vi "6层电梯.vi"() -> ()   [LabVIEW 2014]
panel:
  out "超重灯":bool
  in  "重量":dbl
  in  "常开":bool
  in  "开":bool
  in  "关":bool
  in  "电梯快行":bool
  in  "5下":bool
  out "6楼显示":string
  in  "6下":bool
  out "6楼门":bool
  in  "6楼":bool
  out "电梯内显示":string
  out "5楼显示":string
  out "4楼显示":string
  out "3楼显示":string
  out "2楼显示":string
  out "1楼显示":string
  in  "?":bool
  out "上/下":i32
  in  "2下":bool
  in  "3下":bool
  in  "4下":bool
  in  "3上":bool
  in  "1上":bool
  in  "2上":bool
  in  "4上":bool
  in  "5上":bool
  in  "电梯门":bool
  in  "3楼":bool
  in  "1楼":bool
  in  "2楼":bool
  in  "4楼":bool
  in  "5楼":bool
  out "5楼门":bool
  out "4楼门":bool
  out "3楼门":bool
  out "2楼门":bool
  out "1楼门":bool
  # "门开6秒后检测重量，大于1000则\n不会关门，需手动修改"
  # "模仿人为用物品遮挡电梯门，导致电梯不能\n关门执行下一步动作，常开点亮需手动熄灭\n使电梯门关。"
  # "在门打开期间\n开、关禁止同时点亮，会造成程序运行错误"
  # "点亮开按钮，延时5S关门"
  # "点亮关按钮，门立即关闭"
  # "点亮灯电梯快速运行\n熄灭灯慢速运行"
  # "电梯内按钮"
  # "电梯外部按钮"
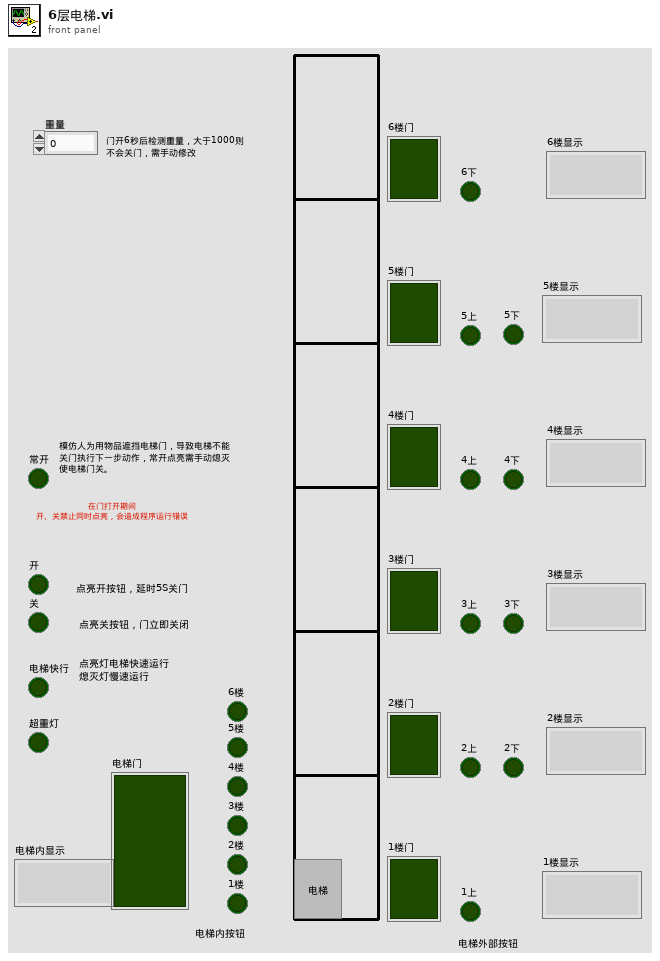
[diagram p1: front panel]
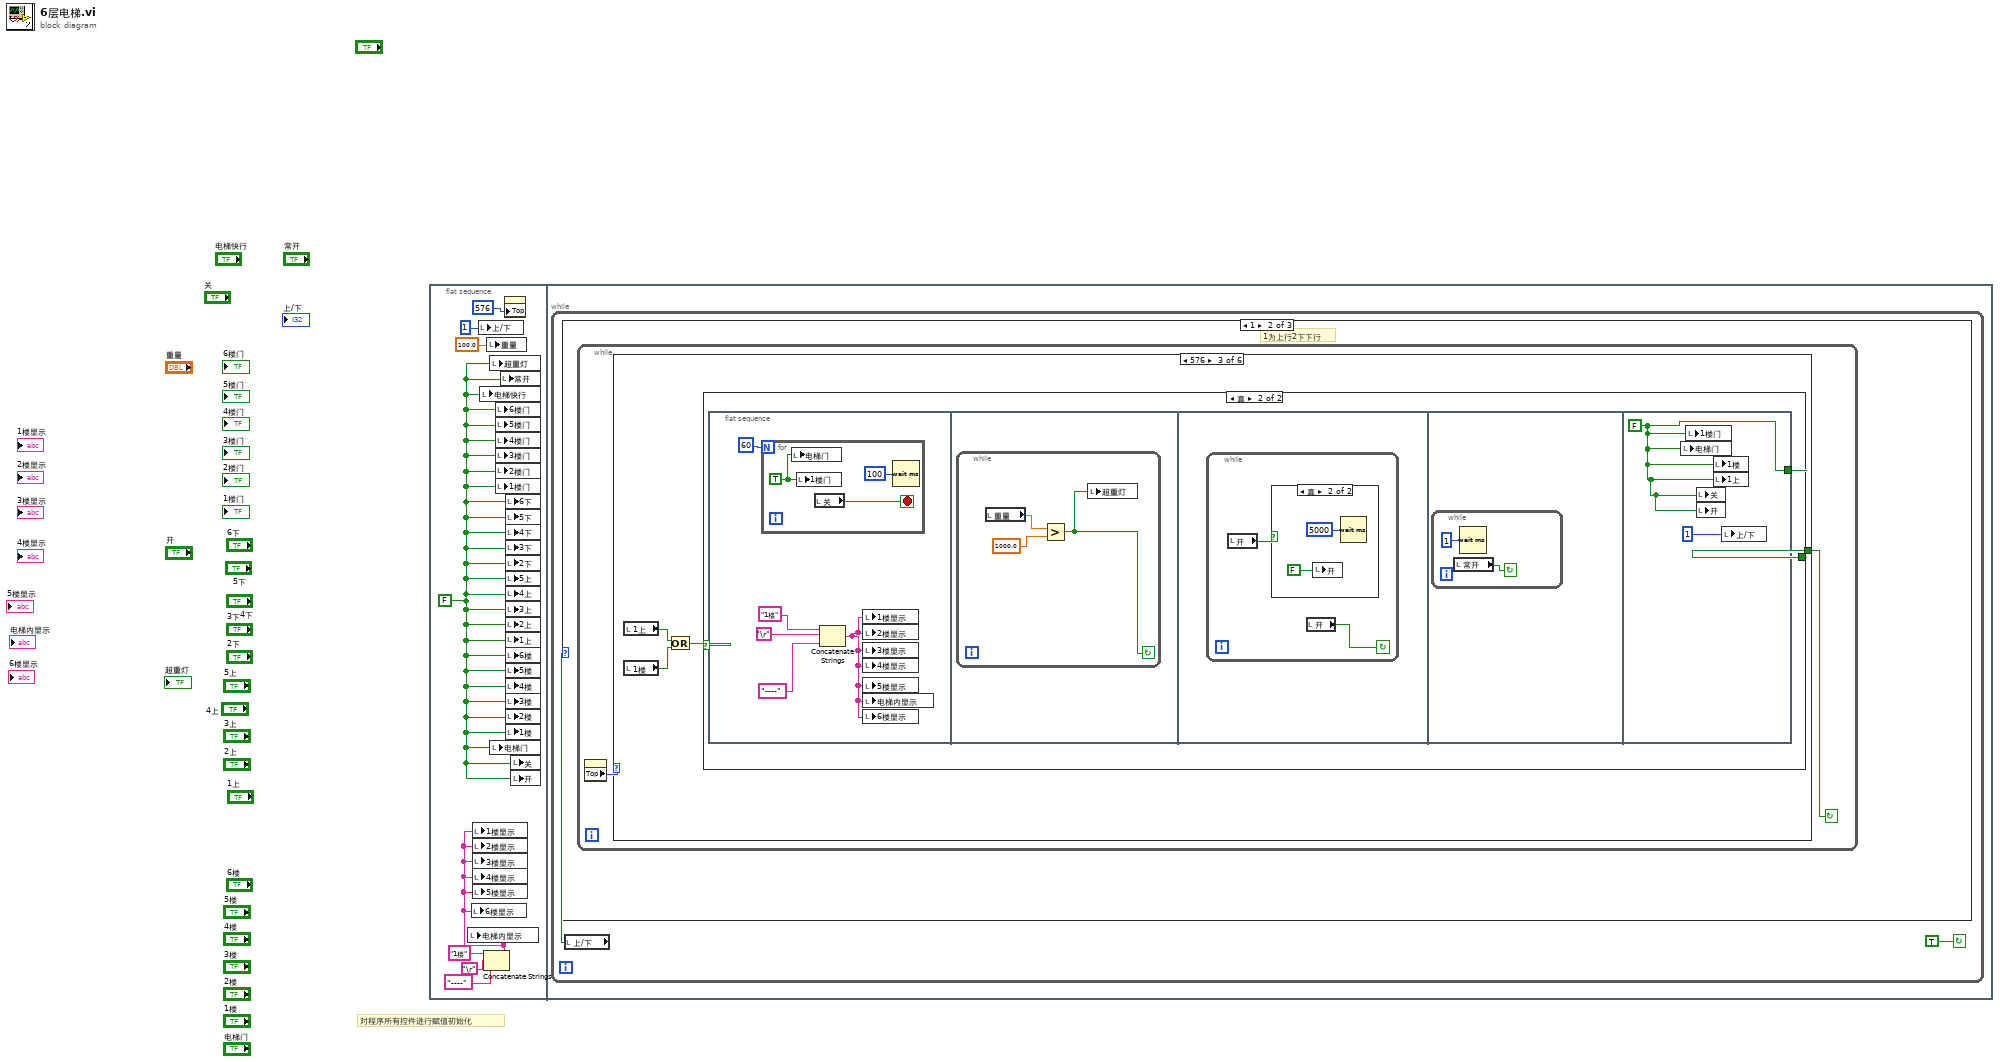
[diagram p0: block diagram]
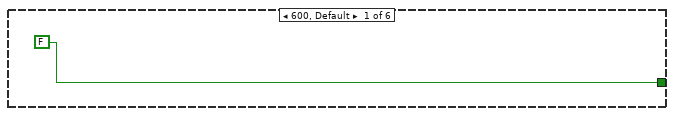
[diagram p3: hidden frame]
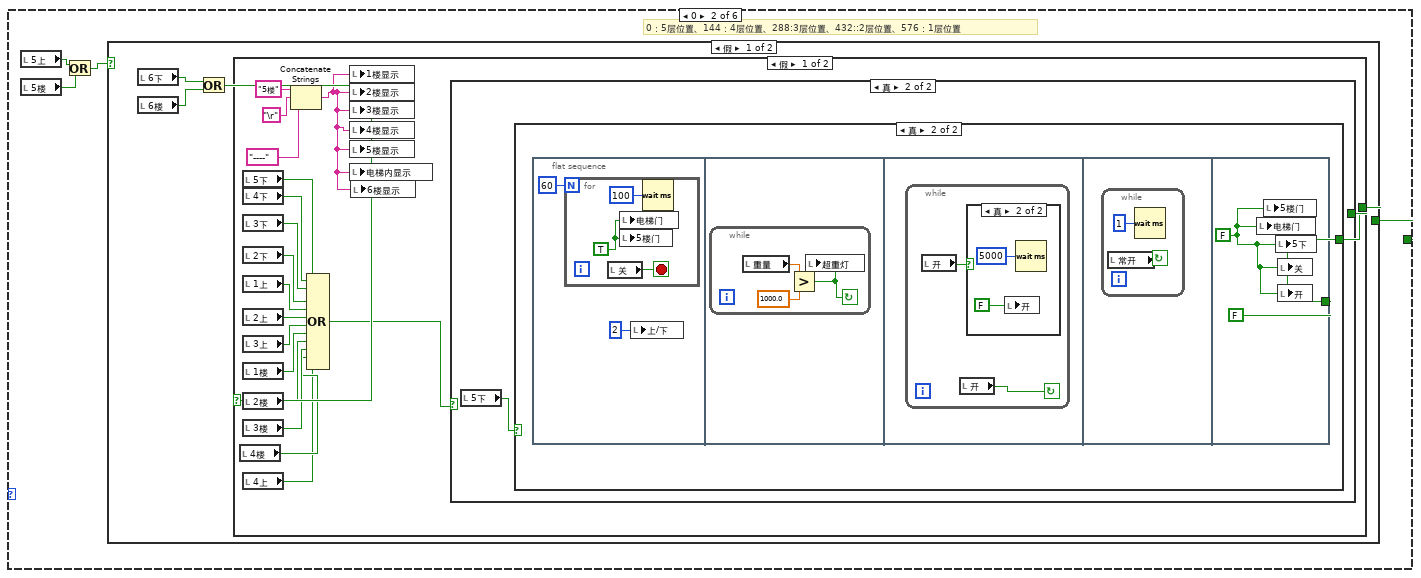
[diagram p4: hidden frame]
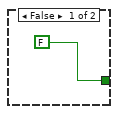
[diagram p5: hidden frame]
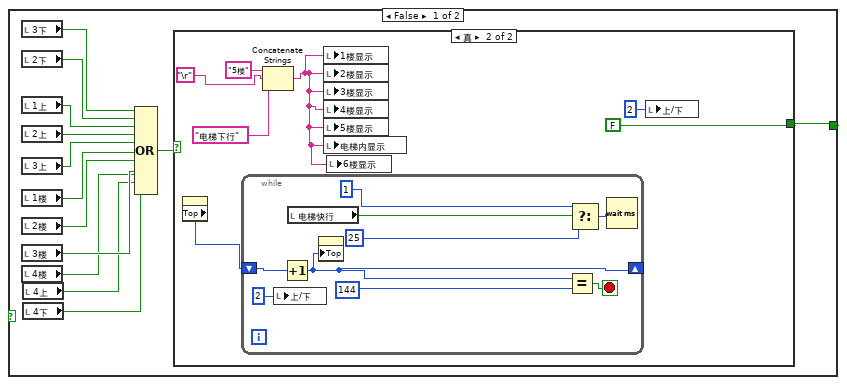
[diagram p6: hidden frame]
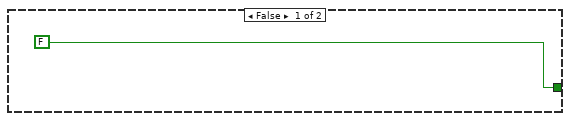
[diagram p7: hidden frame]
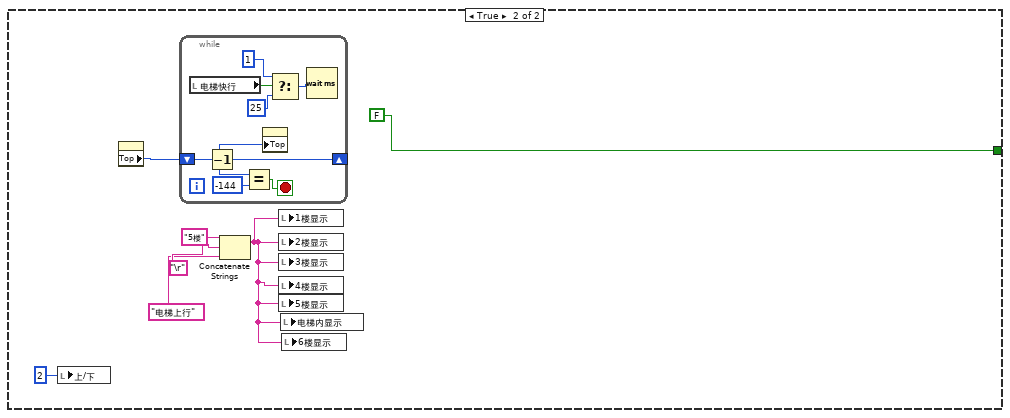
[diagram p9: hidden frame]
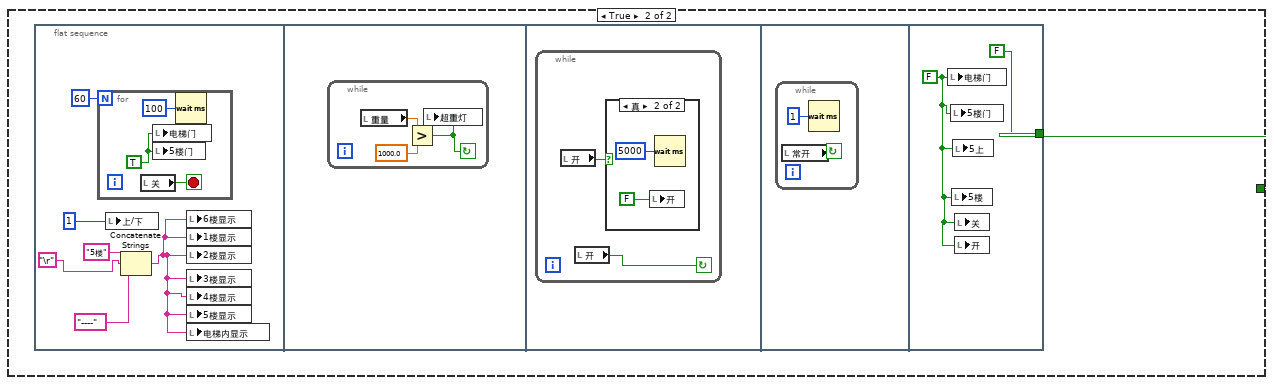
[diagram p10: hidden frame]
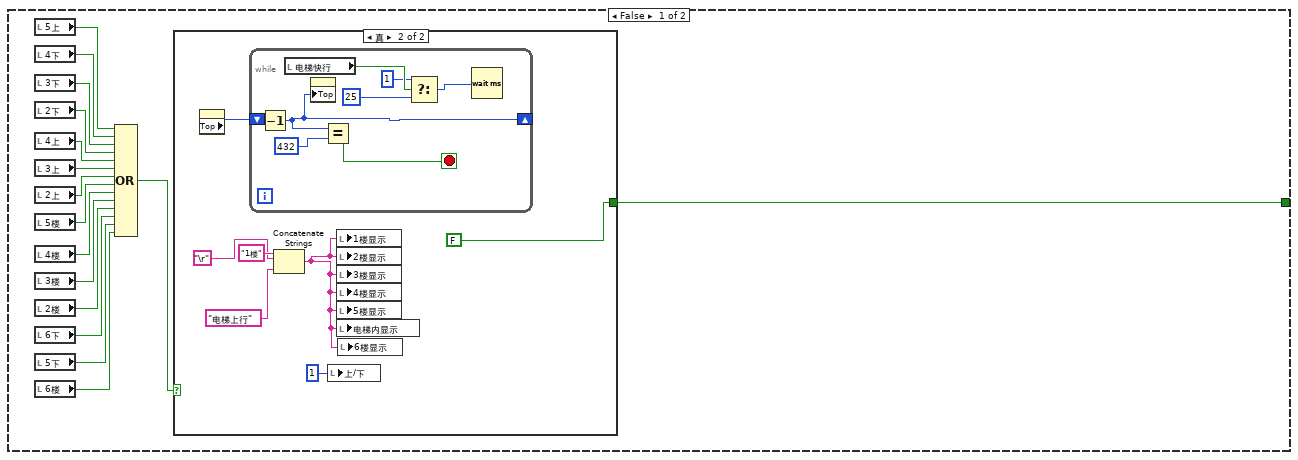
[diagram p12: hidden frame]
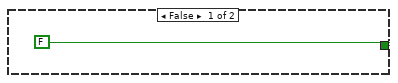
[diagram p13: hidden frame]
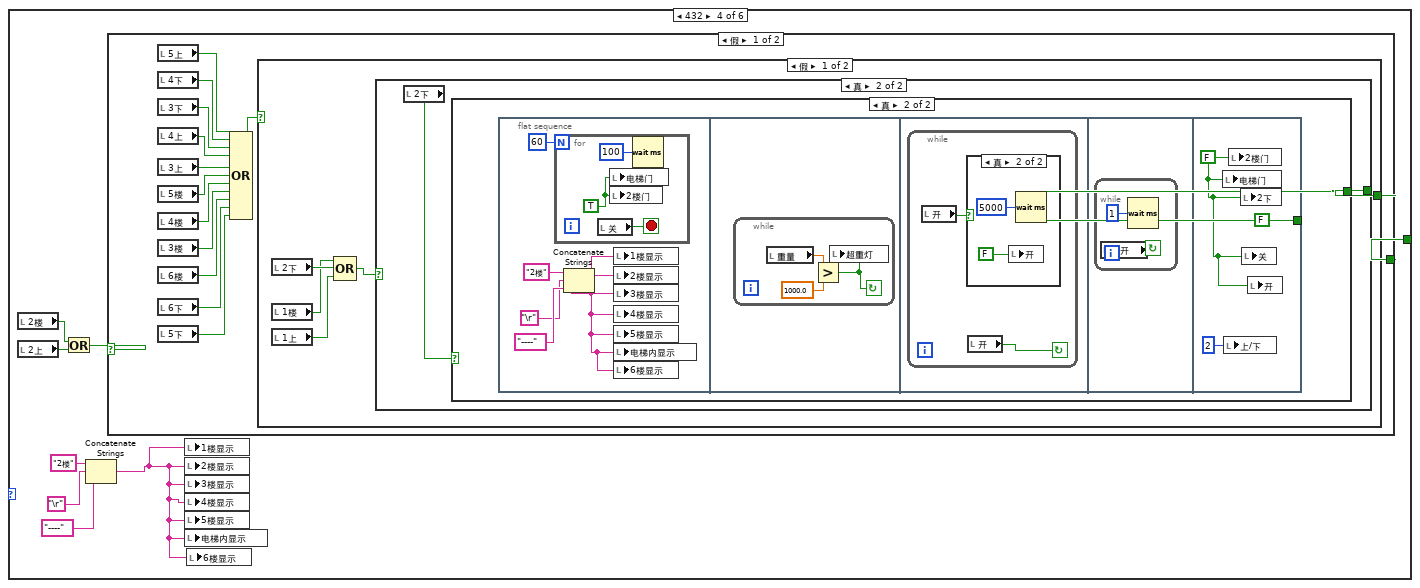
[diagram p15: hidden frame]
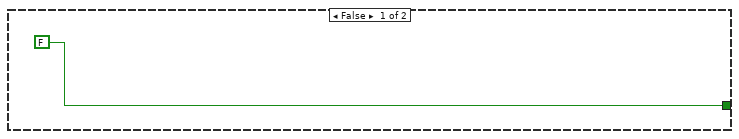
[diagram p16: hidden frame]
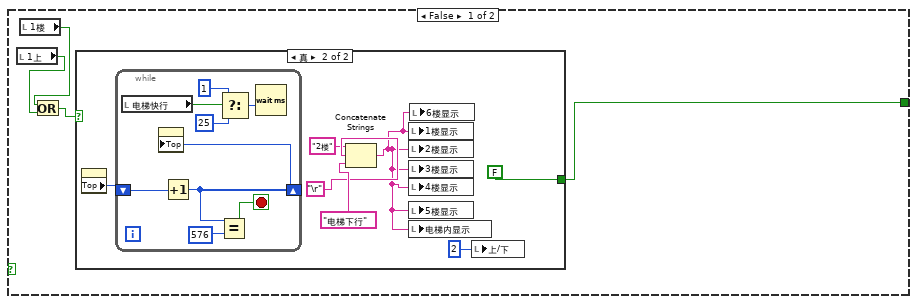
[diagram p17: hidden frame]
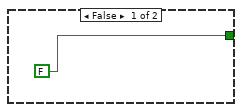
[diagram p18: hidden frame]
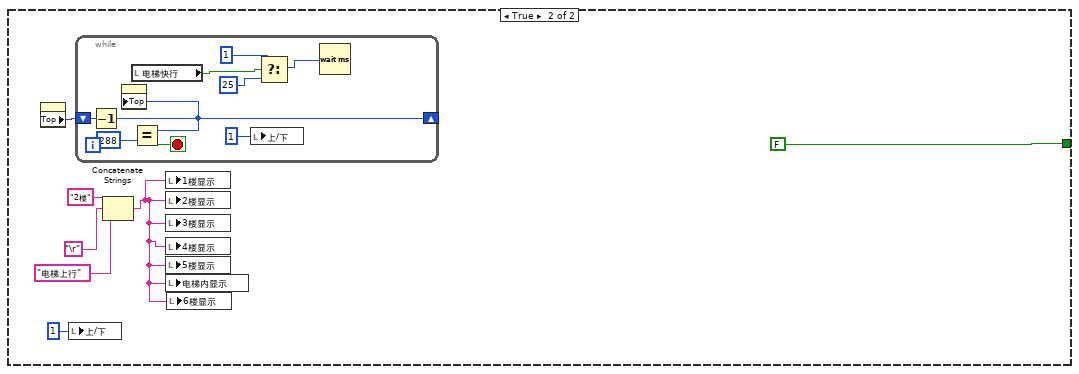
[diagram p20: hidden frame]
diagram:
  # "对程序所有控件进行赋值初始化"
  n1 = flat-sequence {
    frame #0 {
      w1 = FALSE
      n2 = local write "上/下"(1 ("上/下")) -> ()
      n3 = local write "电梯快行"(w1) -> ()
      n4 = Concatenate Strings("1楼" ("字符串"), "\r", "----" ("字符串")) -> (w3:string)
      n5 = local write "电梯内显示"(w3) -> ()
      n6 = local write "6楼显示"(w3) -> ()
      n7 = local write "1楼显示"(w3) -> ()
      n8 = local write "2楼显示"(w3) -> ()
      n9 = local write "3楼显示"(w3) -> ()
      n10 = local write "4楼显示"(w3) -> ()
      n11 = local write "5楼显示"(w3) -> ()
      n12 = local write "重量"(100.0 ("重量")) -> ()
      n13 = local write "超重灯"(w1) -> ()
      n14 = local write "电梯门"(w1) -> ()
      n15 = local write "6楼门"(w1) -> ()
      n16 = local write "5楼门"(w1) -> ()
      n17 = local write "4楼门"(w1) -> ()
      n18 = local write "3楼门"(w1) -> ()
      n19 = local write "2楼门"(w1) -> ()
      n20 = local write "1楼门"(w1) -> ()
      n21 = local write "常开"(w1) -> ()
      n22 = property class="Bool"("Top"=576 ("位置:置顶")) -> ()  [unwired: 2 in, 2 out]
      n23 = local write "6下"(w1) -> ()
      n24 = local write "5下"(w1) -> ()
      n25 = local write "4下"(w1) -> ()
      n26 = local write "3下"(w1) -> ()
      n27 = local write "2下"(w1) -> ()
      n28 = local write "5上"(w1) -> ()
      n29 = local write "4上"(w1) -> ()
      n30 = local write "3上"(w1) -> ()
      n31 = local write "2上"(w1) -> ()
      n32 = local write "1上"(w1) -> ()
      n33 = local write "6楼"(w1) -> ()
      n34 = local write "5楼"(w1) -> ()
      n35 = local write "4楼"(w1) -> ()
      n36 = local write "3楼"(w1) -> ()
      n37 = local write "2楼"(w1) -> ()
      n38 = local write "1楼"(w1) -> ()
      n39 = local write "关"(w1) -> ()
      n40 = local write "开"(w1) -> ()
    }
    frame #1 {
      n41 = while {
        stop <- TRUE continue-if-true
        n42 = local read "上/下"() -> (w10:i32)
        n43 = case shown="1" w10 {
          frame 0, Default {
          }
          frame 1 {
            # "1为上行2下下行"
            n44 = while {
              stop <- w12 continue-if-true
              n45 = property class="Bool"() -> ("Top"=w11:i32)  [unwired: 2 in, 2 out]
              n46 = case shown="576" w11 {
                tunnel: [FALSE w14 w126 w186 w286 w390] -> w12
                frame 600, Default {
                }
                frame 0 {
                  # "0：5层位置、144：4层位置、288:3层位置、432::2层位置、576：1层位置"
                  n47 = local read "5上"() -> (w15:bool)
                  n48 = local read "5楼"() -> (w16:bool)
                  n49 = Or(x=w15, y=w16) -> (x .or. y?=w17:bool)
                  n50 = case shown="假" w17 {
                    tunnel: [w21 w105] -> w14
                    frame False {
                      n51 = local read "6下"() -> (w19:bool)
                      n52 = local read "6楼"() -> (w18:bool)
                      n53 = Or(x=w19, y=w18) -> (x .or. y?=w20:bool)
                      n54 = case shown="假" w20 {
                        tunnel: [w39 FALSE] -> w21
                        frame False {
                          n55 = local read "4楼"() -> (w23:bool)
                          n56 = local read "5下"() -> (w25:bool)
                          n57 = local read "4下"() -> (w35:bool)
                          n58 = local read "3下"() -> (w34:bool)
                          n59 = local read "2下"() -> (w33:bool)
                          n60 = local read "1上"() -> (w32:bool)
                          n61 = local read "2上"() -> (w31:bool)
                          n62 = local read "3上"() -> (w30:bool)
                          n63 = local read "1楼"() -> (w29:bool)
                          n64 = local read "2楼"() -> (w28:bool)
                          n65 = local read "3楼"() -> (w27:bool)
                          n66 = local read "4上"() -> (w22:bool)
                          n67 = Concatenate Strings("5楼" ("字符串"), "\r", "----" ("字符串")) -> (w24:string)
                          n68 = Compound Arithmetic op=OR(w25, w35, w34, w33, w32, w31, w30, w29, w28, w27, w23, w22) -> (w26:bool)
                          n69 = local write "1楼显示"(w24) -> ()
                          n70 = local write "2楼显示"(w24) -> ()
                          n71 = local write "3楼显示"(w24) -> ()
                          n72 = local write "4楼显示"(w24) -> ()
                          n73 = local write "5楼显示"(w24) -> ()
                          n74 = local write "电梯内显示"(w24) -> ()
                          n75 = local write "6楼显示"(w24) -> ()
                          n76 = case shown="真" w26 {
                            tunnel: [FALSE w42] -> w39
                            frame False {
                            }
                            frame True {
                              n77 = local read "5下"() -> (w41:bool)
                              n78 = case shown="真" w41 {
                                tunnel: [w46 w73] -> w42
                                frame False {
                                n79 = local read "3下"() -> (w55:bool)
                                n80 = local read "2下"() -> (w54:bool)
                                n81 = local read "1上"() -> (w53:bool)
                                n82 = local read "2上"() -> (w52:bool)
                                n83 = local read "3上"() -> (w51:bool)
                                n84 = local read "1楼"() -> (w50:bool)
                                n85 = local read "2楼"() -> (w49:bool)
                                n86 = local read "3楼"() -> (w48:bool)
                                n87 = local read "4楼"() -> (w45:bool)
                                n88 = local read "4上"() -> (w44:bool)
                                n89 = local read "4下"() -> (w43:bool)
                                n90 = Compound Arithmetic op=OR(w55, w54, w53, w52, w51, w50, w49, w48, w45, w44, w43) -> (w47:bool)
                                n91 = case shown="真" w47 {
                                tunnel: [FALSE FALSE] -> w46
                                frame False {
                                }
                                frame True {
                                n92 = property class="Bool"() -> ("Top"=w63:i32)  [unwired: 2 in, 2 out]
                                n93 = while {
                                shift-right: [w70] -> _
                                shift-left: w63 -> [w72]
                                stop <- w71 stop-if-true
                                n94 = local write "上/下"(2 ("上/下")) -> ()
                                n95 = Increment(x=w72) -> (x+1=w70:i32)
                                n96 = local read "电梯快行"() -> (w66:bool)
                                n97 = property class="Bool"("Top"=w70) -> ()  [unwired: 2 in, 2 out]
                                n98 = Equal?(x=w70, y=144) -> (x = y?=w71:bool)
                                n99 = Select(t=u32 1, s=w66, f=u32 25) -> (s? t:f=w67:u32)
                                n100 = Wait (ms)(milliseconds to wait=w67) -> ()  [unwired: 1 out]
                                }
                                n101 = Concatenate Strings("5楼" ("字符串"), "\r", "电梯下行" ("字符串")) -> (w57:string)
                                n102 = local write "1楼显示"(w57) -> ()
                                n103 = local write "2楼显示"(w57) -> ()
                                n104 = local write "3楼显示"(w57) -> ()
                                n105 = local write "4楼显示"(w57) -> ()
                                n106 = local write "5楼显示"(w57) -> ()
                                n107 = local write "电梯内显示"(w57) -> ()
                                n108 = local write "6楼显示"(w57) -> ()
                                n109 = local write "上/下"(2 ("上/下")) -> ()
                                }
                                }
                                }
                                frame True {
                                n110 = flat-sequence {
                                tunnel: [FALSE] -> w73
                                frame #0 {
                                n111 = for {
                                N: 60 -> [_]
                                stop <- w76 stop-if-true
                                w78 = TRUE ("1楼门")
                                n112 = local read "关"() -> (w76:bool)
                                n113 = local write "电梯门"(w78) -> ()
                                n114 = local write "5楼门"(w78) -> ()
                                n115 = Wait (ms)(milliseconds to wait=u32 100 ("等待时间（毫秒）")) -> ()  [unwired: 1 out]
                                }
                                n116 = local write "上/下"(2 ("上/下")) -> ()
                                }
                                frame #1 {
                                n117 = while {
                                stop <- w79 continue-if-true
                                n118 = local read "重量"() -> (w81:dbl)
                                n119 = Greater?(x=w81, y=1000.0 ("x")) -> (0:w79:bool)
                                n120 = local write "超重灯"(w79) -> ()
                                }
                                }
                                frame #2 {
                                n121 = while {
                                stop <- w82 continue-if-true
                                n122 = local read "开"() -> (w83:bool)
                                n123 = local read "开"() -> (w82:bool)
                                n124 = case shown="真" w83 {
                                frame False {
                                }
                                frame True {
                                n125 = local write "开"(FALSE ("常开")) -> ()
                                n126 = Wait (ms)(milliseconds to wait=u32 5000 ("等待时间（毫秒）")) -> ()  [unwired: 1 out]
                                }
                                }
                                }
                                }
                                frame #3 {
                                n127 = while {
                                stop <- w87 continue-if-true
                                n128 = local read "常开"() -> (w87:bool)
                                n129 = Wait (ms)(milliseconds to wait=u32 1 ("等待时间（毫秒）")) -> ()  [unwired: 1 out]
                                }
                                }
                                frame #4 {
                                w88 = FALSE ("2楼门")
                                n130 = local write "电梯门"(w88) -> ()
                                n131 = local write "5楼门"(w88) -> ()
                                n132 = local write "5下"(w88) -> ()
                                n133 = local write "关"(w88) -> ()
                                n134 = local write "开"(w88) -> ()
                                }
                                }
                                }
                              }
                            }
                          }
                        }
                        frame True {
                          n135 = local write "上/下"(2 ("上/下")) -> ()
                          n136 = property class="Bool"() -> ("Top"=w90:i32)  [unwired: 2 in, 2 out]
                          n137 = while {
                            shift-right: [w103] -> _
                            shift-left: w90 -> [w101]
                            stop <- w104 stop-if-true
                            n138 = local read "电梯快行"() -> (w99:bool)
                            n139 = Decrement(x=w101) -> (x-1=w103:i32)
                            n140 = Equal?(x=w103, y=-144) -> (x = y?=w104:bool)
                            n141 = property class="Bool"("Top"=w103) -> ()  [unwired: 2 in, 2 out]
                            n142 = Select(t=u32 1, s=w99, f=u32 25) -> (s? t:f=w100:u32)
                            n143 = Wait (ms)(milliseconds to wait=w100) -> ()  [unwired: 1 out]
                          }
                          n144 = Concatenate Strings("5楼" ("字符串"), "\r", "电梯上行" ("字符串")) -> (w94:string)
                          n145 = local write "1楼显示"(w94) -> ()
                          n146 = local write "2楼显示"(w94) -> ()
                          n147 = local write "3楼显示"(w94) -> ()
                          n148 = local write "4楼显示"(w94) -> ()
                          n149 = local write "5楼显示"(w94) -> ()
                          n150 = local write "电梯内显示"(w94) -> ()
                          n151 = local write "6楼显示"(w94) -> ()
                        }
                      }
                    }
                    frame True {
                      n152 = flat-sequence {
                        tunnel: [FALSE] -> w105
                        frame #0 {
                          n153 = for {
                            N: 60 -> [_]
                            stop <- w112 stop-if-true
                            w114 = TRUE ("1楼门")
                            n154 = local read "关"() -> (w112:bool)
                            n155 = local write "电梯门"(w114) -> ()
                            n156 = local write "5楼门"(w114) -> ()
                            n157 = Wait (ms)(milliseconds to wait=u32 100 ("等待时间（毫秒）")) -> ()  [unwired: 1 out]
                          }
                          n158 = local write "上/下"(1 ("上/下")) -> ()
                          n159 = Concatenate Strings("5楼" ("字符串"), "\r", "----" ("字符串")) -> (w107:string)
                          n160 = local write "6楼显示"(w107) -> ()
                          n161 = local write "1楼显示"(w107) -> ()
                          n162 = local write "2楼显示"(w107) -> ()
                          n163 = local write "3楼显示"(w107) -> ()
                          n164 = local write "4楼显示"(w107) -> ()
                          n165 = local write "5楼显示"(w107) -> ()
                          n166 = local write "电梯内显示"(w107) -> ()
                        }
                        frame #1 {
                          n167 = while {
                            stop <- w115 continue-if-true
                            n168 = local read "重量"() -> (w117:dbl)
                            n169 = Greater?(x=w117, y=1000.0 ("x")) -> (0:w115:bool)
                            n170 = local write "超重灯"(w115) -> ()
                          }
                        }
                        frame #2 {
                          n171 = while {
                            stop <- w118 continue-if-true
                            n172 = local read "开"() -> (w119:bool)
                            n173 = local read "开"() -> (w118:bool)
                            n174 = case shown="真" w119 {
                              frame False {
                              }
                              frame True {
                                n175 = local write "开"(FALSE ("常开")) -> ()
                                n176 = Wait (ms)(milliseconds to wait=u32 5000 ("等待时间（毫秒）")) -> ()  [unwired: 1 out]
                              }
                            }
                          }
                        }
                        frame #3 {
                          n177 = while {
                            stop <- w123 continue-if-true
                            n178 = local read "常开"() -> (w123:bool)
                            n179 = Wait (ms)(milliseconds to wait=u32 1 ("等待时间（毫秒）")) -> ()  [unwired: 1 out]
                          }
                        }
                        frame #4 {
                          w124 = FALSE ("电梯门")
                          n180 = local write "电梯门"(w124) -> ()
                          n181 = local write "5楼门"(w124) -> ()
                          n182 = local write "5楼"(w124) -> ()
                          n183 = local write "5上"(w124) -> ()
                          n184 = local write "关"(w124) -> ()
                          n185 = local write "开"(w124) -> ()
                        }
                      }
                    }
                  }
                }
                frame 576 {
                  n186 = local read "1上"() -> (w129:bool)
                  n187 = local read "1楼"() -> (w128:bool)
                  n188 = Or(x=w129, y=w128) -> (x .or. y?=w127:bool)
                  n189 = case shown="真" w127 {
                    tunnel: [w134 w162] -> w126
                    frame False {
                      n190 = local read "5上"() -> (w145:bool)
                      n191 = local read "4下"() -> (w144:bool)
                      n192 = local read "3下"() -> (w143:bool)
                      n193 = local read "2下"() -> (w142:bool)
                      n194 = local read "4上"() -> (w141:bool)
                      n195 = local read "3上"() -> (w140:bool)
                      n196 = local read "2上"() -> (w139:bool)
                      n197 = local read "5楼"() -> (w138:bool)
                      n198 = local read "4楼"() -> (w137:bool)
                      n199 = local read "3楼"() -> (w136:bool)
                      n200 = local read "2楼"() -> (w133:bool)
                      n201 = local read "6下"() -> (w132:bool)
                      n202 = local read "5下"() -> (w131:bool)
                      n203 = local read "6楼"() -> (w130:bool)
                      n204 = Compound Arithmetic op=OR(w145, w144, w143, w142, w141, w140, w139, w138, w137, w136, w133, w132, w131, w130) -> (w135:bool)
                      n205 = case shown="真" w135 {
                        tunnel: [FALSE FALSE] -> w134
                        frame False {
                        }
                        frame True {
                          n206 = property class="Bool"() -> ("Top"=w150:i32)  [unwired: 2 in, 2 out]
                          n207 = while {
                            shift-right: [w159] -> _
                            shift-left: w150 -> [w161]
                            stop <- w160 stop-if-true
                            n208 = Decrement(x=w161) -> (x-1=w159:i32)
                            n209 = local read "电梯快行"() -> (w155:bool)
                            n210 = property class="Bool"("Top"=w159) -> ()  [unwired: 2 in, 2 out]
                            n211 = Equal?(x=w159, y=432) -> (x = y?=w160:bool)
                            n212 = Select(t=u32 1, s=w155, f=u32 25 ("等待时间（毫秒）")) -> (s? t:f=w157:u32)
                            n213 = Wait (ms)(milliseconds to wait=w157) -> ()  [unwired: 1 out]
                          }
                          n214 = Concatenate Strings("1楼" ("字符串"), "\r", "电梯上行" ("字符串")) -> (w147:string)
                          n215 = local write "上/下"(1 ("上/下")) -> ()
                          n216 = local write "1楼显示"(w147) -> ()
                          n217 = local write "2楼显示"(w147) -> ()
                          n218 = local write "3楼显示"(w147) -> ()
                          n219 = local write "4楼显示"(w147) -> ()
                          n220 = local write "5楼显示"(w147) -> ()
                          n221 = local write "电梯内显示"(w147) -> ()
                          n222 = local write "6楼显示"(w147) -> ()
                        }
                      }
                    }
                    frame True {
                      n223 = flat-sequence {
                        tunnel: [w180] -> w162
                        frame #0 {
                          n224 = for {
                            N: 60 -> [_]
                            stop <- w168 stop-if-true
                            w170 = TRUE ("1楼门")
                            n225 = local write "电梯门"(w170) -> ()
                            n226 = local write "1楼门"(w170) -> ()
                            n227 = local read "关"() -> (w168:bool)
                            n228 = Wait (ms)(milliseconds to wait=u32 100 ("等待时间（毫秒）")) -> ()  [unwired: 1 out]
                          }
                          n229 = Concatenate Strings("1楼" ("字符串"), "\r", "----" ("字符串")) -> (w164:string)
                          n230 = local write "1楼显示"(w164) -> ()
                          n231 = local write "2楼显示"(w164) -> ()
                          n232 = local write "3楼显示"(w164) -> ()
                          n233 = local write "4楼显示"(w164) -> ()
                          n234 = local write "5楼显示"(w164) -> ()
                          n235 = local write "电梯内显示"(w164) -> ()
                          n236 = local write "6楼显示"(w164) -> ()
                        }
                        frame #1 {
                          n237 = while {
                            stop <- w171 continue-if-true
                            n238 = local read "重量"() -> (w173:dbl)
                            n239 = Greater?(x=w173, y=1000.0 ("x")) -> (0:w171:bool)
                            n240 = local write "超重灯"(w171) -> ()
                          }
                        }
                        frame #2 {
                          n241 = while {
                            stop <- w174 continue-if-true
                            n242 = local read "开"() -> (w175:bool)
                            n243 = case shown="真" w175 {
                              frame False {
                              }
                              frame True {
                                n244 = local write "开"(FALSE ("常开")) -> ()
                                n245 = Wait (ms)(milliseconds to wait=u32 5000 ("等待时间（毫秒）")) -> ()  [unwired: 1 out]
                              }
                            }
                            n246 = local read "开"() -> (w174:bool)
                          }
                        }
                        frame #3 {
                          n247 = while {
                            stop <- w179 continue-if-true
                            n248 = local read "常开"() -> (w179:bool)
                            n249 = Wait (ms)(milliseconds to wait=u32 1 ("等待时间（毫秒）")) -> ()  [unwired: 1 out]
                          }
                        }
                        frame #4 {
                          w180 = FALSE ("1楼门")
                          n250 = local write "电梯门"(w180) -> ()
                          n251 = local write "1楼门"(w180) -> ()
                          n252 = local write "关"(w180) -> ()
                          n253 = local write "开"(w180) -> ()
                          n254 = local write "1楼"(w180) -> ()
                          n255 = local write "1上"(w180) -> ()
                          n256 = local write "上/下"(1 ("上/下")) -> ()
                        }
                      }
                    }
                  }
                }
                frame 432 {
                  n257 = local read "2楼"() -> (w189:bool)
                  n258 = local read "2上"() -> (w188:bool)
                  n259 = Or(x=w189, y=w188) -> (x .or. y?=w187:bool)
                  n260 = Concatenate Strings("2楼" ("字符串"), "\r", "----" ("字符串")) -> (w182:string)
                  n261 = case shown="假" w187 {
                    tunnel: [w202 w268] -> w186
                    frame False {
                      n262 = local read "5上"() -> (w200:bool)
                      n263 = local read "4下"() -> (w199:bool)
                      n264 = local read "3下"() -> (w198:bool)
                      n265 = local read "4上"() -> (w197:bool)
                      n266 = local read "3上"() -> (w196:bool)
                      n267 = local read "5楼"() -> (w195:bool)
                      n268 = local read "4楼"() -> (w194:bool)
                      n269 = local read "3楼"() -> (w193:bool)
                      n270 = local read "6楼"() -> (w192:bool)
                      n271 = local read "6下"() -> (w191:bool)
                      n272 = local read "5下"() -> (w190:bool)
                      n273 = Compound Arithmetic op=OR(w200, w199, w198, w197, w196, w195, w194, w193, w192, w191, w190) -> (w201:bool)
                      n274 = case shown="假" w201 {
                        tunnel: [w207 FALSE] -> w202
                        frame False {
                          n275 = local read "2下"() -> (w206:bool)
                          n276 = local read "1楼"() -> (w205:bool)
                          n277 = local read "1上"() -> (w204:bool)
                          n278 = Compound Arithmetic op=OR(w205, w206, w204) -> (w203:bool)
                          n279 = case shown="真" w203 {
                            tunnel: [FALSE w210] -> w207
                            frame False {
                            }
                            frame True {
                              n280 = local read "2下"() -> (w209:bool)
                              n281 = case shown="真" w209 {
                                tunnel: [w212 w231] -> w210
                                frame False {
                                n282 = local read "1上"() -> (w213:bool)
                                n283 = local read "1楼"() -> (w214:bool)
                                n284 = Or(x=w214, y=w213) -> (x .or. y?=w211:bool)
                                n285 = case shown="真" w211 {
                                tunnel: [FALSE FALSE] -> w212
                                frame False {
                                }
                                frame True {
                                n286 = property class="Bool"() -> ("Top"=w222:i32)  [unwired: 2 in, 2 out]
                                n287 = while {
                                shift-right: [w228] -> _
                                shift-left: w222 -> [w230]
                                stop <- w229 stop-if-true
                                n288 = local read "电梯快行"() -> (w225:bool)
                                n289 = Increment(x=w230) -> (x+1=w228:i32)
                                n290 = property class="Bool"("Top"=w228) -> ()  [unwired: 2 in, 2 out]
                                n291 = Equal?(x=w228, y=576) -> (x = y?=w229:bool)
                                n292 = Select(t=u32 1, s=w225, f=u32 25 ("等待时间（毫秒）")) -> (s? t:f=w223:u32)
                                n293 = Wait (ms)(milliseconds to wait=w223) -> ()  [unwired: 1 out]
                                }
                                n294 = Concatenate Strings("2楼" ("字符串"), "\r", "电梯下行" ("字符串")) -> (w216:string)
                                n295 = local write "1楼显示"(w216) -> ()
                                n296 = local write "2楼显示"(w216) -> ()
                                n297 = local write "3楼显示"(w216) -> ()
                                n298 = local write "4楼显示"(w216) -> ()
                                n299 = local write "5楼显示"(w216) -> ()
                                n300 = local write "电梯内显示"(w216) -> ()
                                n301 = local write "6楼显示"(w216) -> ()
                                n302 = local write "上/下"(2 ("上/下")) -> ()
                                }
                                }
                                }
                                frame True {
                                n303 = flat-sequence {
                                tunnel: [FALSE] -> w231
                                frame #0 {
                                n304 = for {
                                N: 60 -> [_]
                                stop <- w237 stop-if-true
                                w239 = TRUE ("1楼门")
                                n305 = local read "关"() -> (w237:bool)
                                n306 = local write "电梯门"(w239) -> ()
                                n307 = local write "2楼门"(w239) -> ()
                                n308 = Wait (ms)(milliseconds to wait=u32 100 ("等待时间（毫秒）")) -> ()  [unwired: 1 out]
                                }
                                n309 = Concatenate Strings("2楼" ("字符串"), "\r", "----" ("字符串")) -> (w233:string)
                                n310 = local write "1楼显示"(w233) -> ()
                                n311 = local write "2楼显示"(w233) -> ()
                                n312 = local write "3楼显示"(w233) -> ()
                                n313 = local write "4楼显示"(w233) -> ()
                                n314 = local write "5楼显示"(w233) -> ()
                                n315 = local write "电梯内显示"(w233) -> ()
                                n316 = local write "6楼显示"(w233) -> ()
                                }
                                frame #1 {
                                n317 = while {
                                stop <- w240 continue-if-true
                                n318 = local read "重量"() -> (w242:dbl)
                                n319 = Greater?(x=w242, y=1000.0 ("x")) -> (0:w240:bool)
                                n320 = local write "超重灯"(w240) -> ()
                                }
                                }
                                frame #2 {
                                n321 = while {
                                stop <- w243 continue-if-true
                                n322 = local read "开"() -> (w244:bool)
                                n323 = case shown="真" w244 {
                                frame False {
                                }
                                frame True {
                                n324 = local write "开"(FALSE ("常开")) -> ()
                                n325 = Wait (ms)(milliseconds to wait=u32 5000 ("等待时间（毫秒）")) -> ()  [unwired: 1 out]
                                }
                                }
                                n326 = local read "开"() -> (w243:bool)
                                }
                                }
                                frame #3 {
                                n327 = while {
                                stop <- w248 continue-if-true
                                n328 = local read "常开"() -> (w248:bool)
                                n329 = Wait (ms)(milliseconds to wait=u32 1 ("等待时间（毫秒）")) -> ()  [unwired: 1 out]
                                }
                                }
                                frame #4 {
                                w249 = FALSE ("2楼门")
                                n330 = local write "电梯门"(w249) -> ()
                                n331 = local write "上/下"(2 ("上/下")) -> ()
                                n332 = local write "2楼门"(w249) -> ()
                                n333 = local write "2下"(w249) -> ()
                                n334 = local write "关"(w249) -> ()
                                n335 = local write "开"(w249) -> ()
                                }
                                }
                                }
                              }
                            }
                          }
                        }
                        frame True {
                          n336 = property class="Bool"() -> ("Top"=w258:i32)  [unwired: 2 in, 2 out]
                          n337 = local write "上/下"(1 ("上/下")) -> ()
                          n338 = while {
                            shift-right: [w265] -> _
                            shift-left: w258 -> [w267]
                            stop <- w266 stop-if-true
                            n339 = Decrement(x=w267) -> (x-1=w265:i32)
                            n340 = property class="Bool"("Top"=w265) -> ()  [unwired: 2 in, 2 out]
                            n341 = local read "电梯快行"() -> (w261:bool)
                            n342 = Equal?(x=w265, y=288) -> (x = y?=w266:bool)
                            n343 = local write "上/下"(1 ("上/下")) -> ()
                            n344 = Select(t=u32 1, s=w261, f=u32 25 ("等待时间（毫秒）")) -> (s? t:f=w262:u32)
                            n345 = Wait (ms)(milliseconds to wait=w262) -> ()  [unwired: 1 out]
                          }
                          n346 = Concatenate Strings("2楼" ("字符串"), "\r", "电梯上行" ("字符串")) -> (w252:string)
                          n347 = local write "1楼显示"(w252) -> ()
                          n348 = local write "2楼显示"(w252) -> ()
                          n349 = local write "3楼显示"(w252) -> ()
                          n350 = local write "4楼显示"(w252) -> ()
                          n351 = local write "5楼显示"(w252) -> ()
                          n352 = local write "电梯内显示"(w252) -> ()
                          n353 = local write "6楼显示"(w252) -> ()
                        }
                      }
                    }
                    frame True {
                      n354 = flat-sequence {
                        tunnel: [FALSE] -> w268
                        frame #0 {
                          n355 = for {
                            N: 60 -> [_]
                            stop <- w271 stop-if-true
                            w273 = TRUE ("1楼门")
                            n356 = local read "关"() -> (w271:bool)
                            n357 = local write "电梯门"(w273) -> ()
                            n358 = local write "2楼门"(w273) -> ()
                            n359 = Wait (ms)(milliseconds to wait=u32 100 ("等待时间（毫秒）")) -> ()  [unwired: 1 out]
                          }
                          n360 = local write "上/下"(1 ("上/下")) -> ()
                        }
                        frame #1 {
                          n361 = while {
                            stop <- w274 continue-if-true
                            n362 = local read "重量"() -> (w276:dbl)
                            n363 = Greater?(x=w276, y=1000.0 ("x")) -> (0:w274:bool)
                            n364 = local write "超重灯"(w274) -> ()
                          }
                        }
                        frame #2 {
                          n365 = while {
                            stop <- w277 continue-if-true
                            n366 = local read "开"() -> (w278:bool)
                            n367 = local read "开"() -> (w277:bool)
                            n368 = case shown="真" w278 {
                              frame False {
                              }
                              frame True {
                                n369 = local write "开"(FALSE ("常开")) -> ()
                                n370 = Wait (ms)(milliseconds to wait=u32 5000 ("等待时间（毫秒）")) -> ()  [unwired: 1 out]
                              }
                            }
                          }
                        }
                        frame #3 {
                          n371 = while {
                            stop <- w282 continue-if-true
                            n372 = local read "常开"() -> (w282:bool)
                            n373 = Wait (ms)(milliseconds to wait=u32 1 ("等待时间（毫秒）")) -> ()  [unwired: 1 out]
                          }
                        }
                        frame #4 {
                          w283 = FALSE ("电梯门")
                          n374 = local write "电梯门"(w283) -> ()
                          n375 = local write "2楼门"(w283) -> ()
                          n376 = local write "2上"(w283) -> ()
                          n377 = local write "2楼"(w283) -> ()
                          n378 = local write "关"(w283) -> ()
                          n379 = local write "开"(w283) -> ()
                        }
                      }
                    }
                  }
                  n380 = local write "1楼显示"(w182) -> ()
                  n381 = local write "2楼显示"(w182) -> ()
                  n382 = local write "3楼显示"(w182) -> ()
                  n383 = local write "4楼显示"(w182) -> ()
                  n384 = local write "5楼显示"(w182) -> ()
                  n385 = local write "电梯内显示"(w182) -> ()
                  n386 = local write "6楼显示"(w182) -> ()
                }
                frame 288 {
                  n387 = local read "3上"() -> (w285:bool)
                  n388 = local read "3楼"() -> (w288:bool)
                  n389 = Or(x=w288, y=w285) -> (x .or. y?=w287:bool)
                  n390 = case shown="假" w287 {
                    tunnel: [w298 w373] -> w286
                    frame False {
                      n391 = local read "5上"() -> (w297:bool)
                      n392 = local read "4下"() -> (w296:bool)
                      n393 = local read "4楼"() -> (w295:bool)
                      n394 = local read "4上"() -> (w294:bool)
                      n395 = local read "5楼"() -> (w292:bool)
                      n396 = local read "6下"() -> (w291:bool)
                      n397 = local read "6楼"() -> (w290:bool)
                      n398 = local read "5下"() -> (w289:bool)
                      n399 = Compound Arithmetic op=OR(w297, w296, w295, w294, w292, w291, w290, w289) -> (w293:bool)
                      n400 = case shown="假" w293 {
                        tunnel: [w306 FALSE] -> w298
                        frame False {
                          n401 = local read "2下"() -> (w304:bool)
                          n402 = local read "1楼"() -> (w302:bool)
                          n403 = local read "2楼"() -> (w301:bool)
                          n404 = local read "2上"() -> (w300:bool)
                          n405 = local read "3下"() -> (w305:bool)
                          n406 = local read "1上"() -> (w303:bool)
                          n407 = Compound Arithmetic op=OR(w305, w304, w303, w302, w301, w300) -> (w299:bool)
                          n408 = case shown="真" w299 {
                            tunnel: [FALSE w308] -> w306
                            frame False {
                            }
                            frame True {
                              n409 = local read "3下"() -> (w309:bool)
                              n410 = case shown="真" w309 {
                                tunnel: [w316 w333] -> w308
                                frame False {
                                n411 = local read "2下"() -> (w311:bool)
                                n412 = local read "1上"() -> (w312:bool)
                                n413 = local read "1楼"() -> (w313:bool)
                                n414 = local read "2楼"() -> (w314:bool)
                                n415 = local read "2上"() -> (w315:bool)
                                n416 = Compound Arithmetic op=OR(w311, w312, w313, w314, w315) -> (w310:bool)
                                n417 = case shown="真" w310 {
                                tunnel: [FALSE FALSE] -> w316
                                frame False {
                                }
                                frame True {
                                n418 = property class="Bool"() -> ("Top"=w319:i32)  [unwired: 2 in, 2 out]
                                n419 = local write "上/下"(2 ("上/下")) -> ()
                                n420 = while {
                                shift-right: [w331] -> _
                                shift-left: w319 -> [w332]
                                stop <- w329 stop-if-true
                                n421 = local read "电梯快行"() -> (w327:bool)
                                n422 = Increment(x=w332) -> (x+1=w331:i32)
                                n423 = Select(t=u32 1, s=w327, f=u32 25) -> (s? t:f=w328:u32)
                                n424 = Equal?(x=w331, y=432) -> (x = y?=w329:bool)
                                n425 = property class="Bool"("Top"=w331) -> ()  [unwired: 2 in, 2 out]
                                n426 = Wait (ms)(milliseconds to wait=w328) -> ()  [unwired: 1 out]
                                }
                                n427 = Concatenate Strings("3楼" ("字符串"), "\r", "电梯下行" ("字符串")) -> (w318:string)
                                n428 = local write "1楼显示"(w318) -> ()
                                n429 = local write "2楼显示"(w318) -> ()
                                n430 = local write "3楼显示"(w318) -> ()
                                n431 = local write "4楼显示"(w318) -> ()
                                n432 = local write "5楼显示"(w318) -> ()
                                n433 = local write "电梯内显示"(w318) -> ()
                                n434 = local write "6楼显示"(w318) -> ()
                                }
                                }
                                }
                                frame True {
                                n435 = flat-sequence {
                                tunnel: [FALSE] -> w333
                                frame #0 {
                                n436 = for {
                                N: 60 -> [_]
                                stop <- w339 stop-if-true
                                w341 = TRUE ("1楼门")
                                n437 = local read "关"() -> (w339:bool)
                                n438 = local write "电梯门"(w341) -> ()
                                n439 = local write "3楼门"(w341) -> ()
                                n440 = Wait (ms)(milliseconds to wait=u32 100 ("等待时间（毫秒）")) -> ()  [unwired: 1 out]
                                }
                                n441 = Concatenate Strings("3楼" ("字符串"), "\r", "----" ("字符串")) -> (w335:string)
                                n442 = local write "电梯内显示"(w335) -> ()
                                n443 = local write "6楼显示"(w335) -> ()
                                n444 = local write "1楼显示"(w335) -> ()
                                n445 = local write "2楼显示"(w335) -> ()
                                n446 = local write "3楼显示"(w335) -> ()
                                n447 = local write "4楼显示"(w335) -> ()
                                n448 = local write "5楼显示"(w335) -> ()
                                }
                                frame #1 {
                                n449 = while {
                                stop <- w342 continue-if-true
                                n450 = local read "重量"() -> (w344:dbl)
                                n451 = Greater?(x=w344, y=1000.0 ("x")) -> (0:w342:bool)
                                n452 = local write "超重灯"(w342) -> ()
                                }
                                }
                                frame #2 {
                                n453 = while {
                                stop <- w345 continue-if-true
                                n454 = local read "开"() -> (w346:bool)
                                n455 = local read "开"() -> (w345:bool)
                                n456 = case shown="真" w346 {
                                frame False {
                                }
                                frame True {
                                n457 = local write "开"(FALSE ("常开")) -> ()
                                n458 = Wait (ms)(milliseconds to wait=u32 5000 ("等待时间（毫秒）")) -> ()  [unwired: 1 out]
                                }
                                }
                                }
                                }
                                frame #3 {
                                n459 = while {
                                stop <- w350 continue-if-true
                                n460 = local read "常开"() -> (w350:bool)
                                n461 = Wait (ms)(milliseconds to wait=u32 1 ("等待时间（毫秒）")) -> ()  [unwired: 1 out]
                                }
                                }
                                frame #4 {
                                w351 = FALSE ("电梯门")
                                n462 = local write "电梯门"(w351) -> ()
                                n463 = local write "3楼门"(w351) -> ()
                                n464 = local write "关"(w351) -> ()
                                n465 = local write "开"(w351) -> ()
                                n466 = local write "3下"(w351) -> ()
                                n467 = local write "3楼"(w351) -> ()
                                n468 = local write "上/下"(2 ("上/下")) -> ()
                                }
                                }
                                }
                              }
                            }
                          }
                        }
                        frame True {
                          n469 = Concatenate Strings("3楼" ("字符串"), "\r", "电梯上行" ("字符串")) -> (w358:string)
                          n470 = local write "上/下"(1 ("上/下")) -> ()
                          n471 = local write "1楼显示"(w358) -> ()
                          n472 = local write "2楼显示"(w358) -> ()
                          n473 = local write "3楼显示"(w358) -> ()
                          n474 = local write "4楼显示"(w358) -> ()
                          n475 = local write "5楼显示"(w358) -> ()
                          n476 = local write "电梯内显示"(w358) -> ()
                          n477 = local write "6楼显示"(w358) -> ()
                          n478 = property class="Bool"() -> ("Top"=w360:i32)  [unwired: 2 in, 2 out]
                          n479 = while {
                            shift-right: [w366] -> _
                            shift-left: w360 -> [w368]
                            stop <- w367 stop-if-true
                            n480 = Decrement(x=w368) -> (x-1=w366:i32)
                            n481 = property class="Bool"("Top"=w366) -> ()  [unwired: 2 in, 2 out]
                            n482 = Equal?(x=w366, y=144) -> (x = y?=w367:bool)
                            n483 = local read "电梯快行"() -> (w363:bool)
                            n484 = Select(t=u32 1, s=w363, f=u32 25) -> (s? t:f=w364:u32)
                            n485 = Wait (ms)(milliseconds to wait=w364) -> ()  [unwired: 1 out]
                          }
                        }
                      }
                    }
                    frame True {
                      n486 = flat-sequence {
                        tunnel: [FALSE] -> w373
                        frame #0 {
                          n487 = for {
                            N: 60 -> [_]
                            stop <- w376 stop-if-true
                            w378 = TRUE ("1楼门")
                            n488 = local read "关"() -> (w376:bool)
                            n489 = local write "电梯门"(w378) -> ()
                            n490 = local write "3楼门"(w378) -> ()
                            n491 = Wait (ms)(milliseconds to wait=u32 100 ("等待时间（毫秒）")) -> ()  [unwired: 1 out]
                          }
                          n492 = local write "上/下"(1 ("上/下")) -> ()
                        }
                        frame #1 {
                          n493 = while {
                            stop <- w379 continue-if-true
                            n494 = local read "重量"() -> (w381:dbl)
                            n495 = Greater?(x=w381, y=1000.0 ("x")) -> (0:w379:bool)
                            n496 = local write "超重灯"(w379) -> ()
                          }
                        }
                        frame #2 {
                          n497 = while {
                            stop <- w382 continue-if-true
                            n498 = local read "开"() -> (w383:bool)
                            n499 = local read "开"() -> (w382:bool)
                            n500 = case shown="真" w383 {
                              frame False {
                              }
                              frame True {
                                n501 = local write "开"(FALSE ("常开")) -> ()
                                n502 = Wait (ms)(milliseconds to wait=u32 5000 ("等待时间（毫秒）")) -> ()  [unwired: 1 out]
                              }
                            }
                          }
                        }
                        frame #3 {
                          n503 = while {
                            stop <- w387 continue-if-true
                            n504 = local read "常开"() -> (w387:bool)
                            n505 = Wait (ms)(milliseconds to wait=u32 1 ("等待时间（毫秒）")) -> ()  [unwired: 1 out]
                          }
                        }
                        frame #4 {
                          w388 = FALSE ("电梯门")
                          n506 = local write "电梯门"(w388) -> ()
                          n507 = local write "3楼门"(w388) -> ()
                          n508 = local write "3上"(w388) -> ()
                          n509 = local write "3楼"(w388) -> ()
                          n510 = local write "开"(w388) -> ()
                          n511 = local write "关"(w388) -> ()
                        }
                      }
                      n512 = Concatenate Strings("3楼" ("字符串"), "\r", "----" ("字符串")) -> (w369:string)
                      n513 = local write "1楼显示"(w369) -> ()
                      n514 = local write "2楼显示"(w369) -> ()
                      n515 = local write "3楼显示"(w369) -> ()
                      n516 = local write "4楼显示"(w369) -> ()
                      n517 = local write "5楼显示"(w369) -> ()
                      n518 = local write "电梯内显示"(w369) -> ()
                      n519 = local write "6楼显示"(w369) -> ()
                    }
                  }
                }
                frame 144 {
                  n520 = local read "4上"() -> (w392:bool)
                  n521 = local read "4楼"() -> (w393:bool)
                  n522 = Or(x=w392, y=w393) -> (x .or. y?=w391:bool)
                  n523 = case shown="假" w391 {
                    tunnel: [w394 w478] -> w390
                    frame False {
                      n524 = local read "5上"() -> (w400:bool)
                      n525 = local read "5楼"() -> (w399:bool)
                      n526 = local read "5下"() -> (w398:bool)
                      n527 = local read "6下"() -> (w397:bool)
                      n528 = local read "6楼"() -> (w396:bool)
                      n529 = Compound Arithmetic op=OR(w400, w399, w398, w397, w396) -> (w395:bool)
                      n530 = case shown="假" w395 {
                        tunnel: [w415 FALSE] -> w394
                        frame False {
                          n531 = local read "4下"() -> (w411:bool)
                          n532 = local read "3下"() -> (w410:bool)
                          n533 = local read "2下"() -> (w409:bool)
                          n534 = local read "1上"() -> (w408:bool)
                          n535 = local read "2上"() -> (w407:bool)
                          n536 = local read "3上"() -> (w406:bool)
                          n537 = local read "1楼"() -> (w405:bool)
                          n538 = local read "2楼"() -> (w404:bool)
                          n539 = local read "3楼"() -> (w403:bool)
                          n540 = Concatenate Strings("4楼" ("字符串"), "\r", "----" ("字符串")) -> (w401:string)
                          n541 = Compound Arithmetic op=OR(w411, w410, w409, w408, w407, w406, w405, w404, w403) -> (w402:bool)
                          n542 = local write "1楼显示"(w401) -> ()
                          n543 = local write "2楼显示"(w401) -> ()
                          n544 = local write "3楼显示"(w401) -> ()
                          n545 = local write "4楼显示"(w401) -> ()
                          n546 = local write "5楼显示"(w401) -> ()
                          n547 = local write "电梯内显示"(w401) -> ()
                          n548 = local write "6楼显示"(w401) -> ()
                          n549 = case shown="真" w402 {
                            tunnel: [FALSE w418] -> w415
                            frame False {
                            }
                            frame True {
                              n550 = local read "4下"() -> (w417:bool)
                              n551 = case shown="真" w417 {
                                tunnel: [w419 w446] -> w418
                                frame False {
                                n552 = local read "3下"() -> (w428:bool)
                                n553 = local read "2下"() -> (w427:bool)
                                n554 = local read "1上"() -> (w426:bool)
                                n555 = local read "2上"() -> (w425:bool)
                                n556 = local read "3上"() -> (w424:bool)
                                n557 = local read "1楼"() -> (w423:bool)
                                n558 = local read "2楼"() -> (w422:bool)
                                n559 = local read "3楼"() -> (w421:bool)
                                n560 = Compound Arithmetic op=OR(w428, w427, w426, w425, w424, w423, w422, w421) -> (w420:bool)
                                n561 = case shown="真" w420 {
                                tunnel: [FALSE FALSE] -> w419
                                frame False {
                                }
                                frame True {
                                n562 = property class="Bool"() -> ("Top"=w436:i32)  [unwired: 2 in, 2 out]
                                n563 = while {
                                shift-right: [w443] -> _
                                shift-left: w436 -> [w445]
                                stop <- w444 stop-if-true
                                n564 = local write "上/下"(2 ("上/下")) -> ()
                                n565 = Increment(x=w445) -> (x+1=w443:i32)
                                n566 = local read "电梯快行"() -> (w439:bool)
                                n567 = property class="Bool"("Top"=w443) -> ()  [unwired: 2 in, 2 out]
                                n568 = Equal?(x=w443, y=288) -> (x = y?=w444:bool)
                                n569 = Select(t=u32 1, s=w439, f=u32 25) -> (s? t:f=w440:u32)
                                n570 = Wait (ms)(milliseconds to wait=w440) -> ()  [unwired: 1 out]
                                }
                                n571 = Concatenate Strings("4楼" ("字符串"), "\r", "电梯下行" ("字符串")) -> (w430:string)
                                n572 = local write "1楼显示"(w430) -> ()
                                n573 = local write "2楼显示"(w430) -> ()
                                n574 = local write "3楼显示"(w430) -> ()
                                n575 = local write "4楼显示"(w430) -> ()
                                n576 = local write "5楼显示"(w430) -> ()
                                n577 = local write "电梯内显示"(w430) -> ()
                                n578 = local write "6楼显示"(w430) -> ()
                                n579 = local write "上/下"(2 ("上/下")) -> ()
                                }
                                }
                                }
                                frame True {
                                n580 = flat-sequence {
                                tunnel: [FALSE] -> w446
                                frame #0 {
                                n581 = for {
                                N: 60 -> [_]
                                stop <- w449 stop-if-true
                                w451 = TRUE ("1楼门")
                                n582 = local read "关"() -> (w449:bool)
                                n583 = local write "电梯门"(w451) -> ()
                                n584 = local write "4楼门"(w451) -> ()
                                n585 = Wait (ms)(milliseconds to wait=u32 100 ("等待时间（毫秒）")) -> ()  [unwired: 1 out]
                                }
                                n586 = local write "上/下"(1 ("上/下")) -> ()
                                }
                                frame #1 {
                                n587 = while {
                                stop <- w452 continue-if-true
                                n588 = local read "重量"() -> (w454:dbl)
                                n589 = Greater?(x=w454, y=1000.0 ("x")) -> (0:w452:bool)
                                n590 = local write "超重灯"(w452) -> ()
                                }
                                }
                                frame #2 {
                                n591 = while {
                                stop <- w455 continue-if-true
                                n592 = local read "开"() -> (w456:bool)
                                n593 = local read "开"() -> (w455:bool)
                                n594 = case shown="真" w456 {
                                frame False {
                                }
                                frame True {
                                n595 = local write "开"(FALSE ("常开")) -> ()
                                n596 = Wait (ms)(milliseconds to wait=u32 5000 ("等待时间（毫秒）")) -> ()  [unwired: 1 out]
                                }
                                }
                                }
                                }
                                frame #3 {
                                n597 = while {
                                stop <- w460 continue-if-true
                                n598 = local read "常开"() -> (w460:bool)
                                n599 = Wait (ms)(milliseconds to wait=u32 1 ("等待时间（毫秒）")) -> ()  [unwired: 1 out]
                                }
                                }
                                frame #4 {
                                w461 = FALSE ("2楼门")
                                n600 = local write "电梯门"(w461) -> ()
                                n601 = local write "4楼门"(w461) -> ()
                                n602 = local write "4下"(w461) -> ()
                                n603 = local write "关"(w461) -> ()
                                n604 = local write "开"(w461) -> ()
                                }
                                }
                                }
                              }
                            }
                          }
                        }
                        frame True {
                          n605 = local write "上/下"(1 ("上/下")) -> ()
                          n606 = property class="Bool"() -> ("Top"=w463:i32)  [unwired: 2 in, 2 out]
                          n607 = while {
                            shift-right: [w474] -> _
                            shift-left: w463 -> [w475]
                            stop <- w477 stop-if-true
                            n608 = Decrement(x=w475) -> (x-1=w474:i32)
                            n609 = Equal?(x=w474, y=0) -> (x = y?=w477:bool)
                            n610 = property class="Bool"("Top"=w474) -> ()  [unwired: 2 in, 2 out]
                            n611 = local read "电梯快行"() -> (w472:bool)
                            n612 = Select(t=u32 1, s=w472, f=u32 25) -> (s? t:f=w473:u32)
                            n613 = Wait (ms)(milliseconds to wait=w473) -> ()  [unwired: 1 out]
                          }
                          n614 = Concatenate Strings("4楼" ("字符串"), "\r", "电梯上行" ("字符串")) -> (w468:string)
                          n615 = local write "1楼显示"(w468) -> ()
                          n616 = local write "2楼显示"(w468) -> ()
                          n617 = local write "3楼显示"(w468) -> ()
                          n618 = local write "4楼显示"(w468) -> ()
                          n619 = local write "5楼显示"(w468) -> ()
                          n620 = local write "电梯内显示"(w468) -> ()
                          n621 = local write "6楼显示"(w468) -> ()
                        }
                      }
                    }
                    frame True {
                      n622 = flat-sequence {
                        tunnel: [FALSE] -> w478
                        frame #0 {
                          n623 = for {
                            N: 60 -> [_]
                            stop <- w485 stop-if-true
                            w487 = TRUE ("1楼门")
                            n624 = local read "关"() -> (w485:bool)
                            n625 = local write "电梯门"(w487) -> ()
                            n626 = local write "4楼门"(w487) -> ()
                            n627 = Wait (ms)(milliseconds to wait=u32 100 ("等待时间（毫秒）")) -> ()  [unwired: 1 out]
                          }
                          n628 = local write "上/下"(1 ("上/下")) -> ()
                          n629 = Concatenate Strings("4楼" ("字符串"), "\r", "----" ("字符串")) -> (w480:string)
                          n630 = local write "6楼显示"(w480) -> ()
                          n631 = local write "1楼显示"(w480) -> ()
                          n632 = local write "2楼显示"(w480) -> ()
                          n633 = local write "3楼显示"(w480) -> ()
                          n634 = local write "4楼显示"(w480) -> ()
                          n635 = local write "5楼显示"(w480) -> ()
                          n636 = local write "电梯内显示"(w480) -> ()
                        }
                        frame #1 {
                          n637 = while {
                            stop <- w488 continue-if-true
                            n638 = local read "重量"() -> (w490:dbl)
                            n639 = Greater?(x=w490, y=1000.0 ("x")) -> (0:w488:bool)
                            n640 = local write "超重灯"(w488) -> ()
                          }
                        }
                        frame #2 {
                          n641 = while {
                            stop <- w491 continue-if-true
                            n642 = local read "开"() -> (w492:bool)
                            n643 = case shown="真" w492 {
                              frame False {
                              }
                              frame True {
                                n644 = local write "开"(FALSE ("常开")) -> ()
                                n645 = Wait (ms)(milliseconds to wait=u32 5000 ("等待时间（毫秒）")) -> ()  [unwired: 1 out]
                              }
                            }
                            n646 = local read "开"() -> (w491:bool)
                          }
                        }
                        frame #3 {
                          n647 = while {
                            stop <- w496 continue-if-true
                            n648 = local read "常开"() -> (w496:bool)
                            n649 = Wait (ms)(milliseconds to wait=u32 1 ("等待时间（毫秒）")) -> ()  [unwired: 1 out]
                          }
                        }
                        frame #4 {
                          w497 = FALSE ("电梯门")
                          n650 = local write "电梯门"(w497) -> ()
                          n651 = local write "4楼门"(w497) -> ()
                          n652 = local write "4上"(w497) -> ()
                          n653 = local write "4楼"(w497) -> ()
                          n654 = local write "开"(w497) -> ()
                          n655 = local write "关"(w497) -> ()
                        }
                      }
                    }
                  }
                }
              }
            }
          }
          frame 2 {
            n656 = while {
              stop <- w499 continue-if-true
              n657 = property class="Bool"() -> ("Top"=w500:i32)  [unwired: 2 in, 2 out]
              n658 = case shown="288" w500 {
                tunnel: [FALSE w502 w625 _ w806 w935] -> w499
                frame 600, Default {
                }
                frame 144 {
                  n659 = local read "4下"() -> (w504:bool)
                  n660 = local read "4楼"() -> (w505:bool)
                  n661 = Or(x=w504, y=w505) -> (x .or. y?=w503:bool)
                  n662 = case shown="真" w503 {
                    tunnel: [w510 w604] -> w502
                    frame False {
                      n663 = local read "5下"() -> (w508:bool)
                      n664 = local read "6楼"() -> (w507:bool)
                      n665 = local read "6下"() -> (w506:bool)
                      n666 = local read "5上"() -> (w521:bool)
                      n667 = local read "1楼"() -> (w520:bool)
                      n668 = local read "3下"() -> (w519:bool)
                      n669 = local read "2下"() -> (w518:bool)
                      n670 = local read "4上"() -> (w517:bool)
                      n671 = local read "3上"() -> (w516:bool)
                      n672 = local read "2上"() -> (w515:bool)
                      n673 = local read "5楼"() -> (w514:bool)
                      n674 = local read "1上"() -> (w513:bool)
                      n675 = local read "3楼"() -> (w512:bool)
                      n676 = local read "2楼"() -> (w509:bool)
                      n677 = Compound Arithmetic op=OR(w521, w520, w519, w518, w517, w516, w515, w514, w513, w512, w509, w508, w507, w506) -> (w511:bool)
                      n678 = case shown="真" w511 {
                        tunnel: [FALSE w532] -> w510
                        frame False {
                        }
                        frame True {
                          n679 = local read "1楼"() -> (w531:bool)
                          n680 = local read "3下"() -> (w530:bool)
                          n681 = local read "2下"() -> (w529:bool)
                          n682 = local read "3上"() -> (w528:bool)
                          n683 = local read "3楼"() -> (w527:bool)
                          n684 = local read "2楼"() -> (w526:bool)
                          n685 = local read "1上"() -> (w524:bool)
                          n686 = local read "2上"() -> (w523:bool)
                          n687 = Compound Arithmetic op=OR(w531, w530, w529, w528, w527, w526, w524, w523) -> (w525:bool)
                          n688 = case shown="假" w525 {
                            tunnel: [w536 w588] -> w532
                            frame False {
                              n689 = local read "5下"() -> (w535:bool)
                              n690 = local read "6下"() -> (w533:bool)
                              n691 = local read "6楼"() -> (w534:bool)
                              n692 = local read "5上"() -> (w540:bool)
                              n693 = local read "4上"() -> (w539:bool)
                              n694 = local read "5楼"() -> (w538:bool)
                              n695 = Compound Arithmetic op=OR(w540, w539, w538, w535, w534, w533) -> (w537:bool)
                              n696 = case shown="真" w537 {
                                tunnel: [FALSE w542] -> w536
                                frame False {
                                }
                                frame True {
                                n697 = local read "4上"() -> (w543:bool)
                                n698 = case shown="真" w543 {
                                tunnel: [w550 w567] -> w542
                                frame False {
                                n699 = local read "5下"() -> (w549:bool)
                                n700 = local read "6下"() -> (w547:bool)
                                n701 = local read "6楼"() -> (w548:bool)
                                n702 = local read "5上"() -> (w546:bool)
                                n703 = local read "5楼"() -> (w545:bool)
                                n704 = Compound Arithmetic op=OR(w549, w548, w547, w546, w545) -> (w544:bool)
                                n705 = case shown="真" w544 {
                                tunnel: [FALSE FALSE] -> w550
                                frame False {
                                }
                                frame True {
                                n706 = property class="Bool"() -> ("Top"=w558:i32)  [unwired: 2 in, 2 out]
                                n707 = while {
                                shift-right: [w564] -> _
                                shift-left: w558 -> [w566]
                                stop <- w565 stop-if-true
                                n708 = local read "电梯快行"() -> (w561:bool)
                                n709 = Decrement(x=w566) -> (x-1=w564:i32)
                                n710 = Select(t=u32 1, s=w561, f=u32 25) -> (s? t:f=w562:u32)
                                n711 = Equal?(x=w564, y=0) -> (x = y?=w565:bool)
                                n712 = property class="Bool"("Top"=w564) -> ()  [unwired: 2 in, 2 out]
                                n713 = Wait (ms)(milliseconds to wait=w562) -> ()  [unwired: 1 out]
                                }
                                n714 = Concatenate Strings("4楼" ("字符串"), "\r", "电梯上行" ("字符串")) -> (w553:string)
                                n715 = local write "1楼显示"(w553) -> ()
                                n716 = local write "2楼显示"(w553) -> ()
                                n717 = local write "3楼显示"(w553) -> ()
                                n718 = local write "4楼显示"(w553) -> ()
                                n719 = local write "5楼显示"(w553) -> ()
                                n720 = local write "电梯内显示"(w553) -> ()
                                n721 = local write "6楼显示"(w553) -> ()
                                n722 = local write "上/下"(1 ("上/下")) -> ()
                                }
                                }
                                }
                                frame True {
                                n723 = flat-sequence {
                                tunnel: [FALSE] -> w567
                                frame #0 {
                                n724 = for {
                                N: 60 -> [_]
                                stop <- w574 stop-if-true
                                w576 = TRUE ("1楼门")
                                n725 = local read "关"() -> (w574:bool)
                                n726 = local write "电梯门"(w576) -> ()
                                n727 = local write "4楼门"(w576) -> ()
                                n728 = Wait (ms)(milliseconds to wait=u32 100 ("等待时间（毫秒）")) -> ()  [unwired: 1 out]
                                }
                                n729 = local write "上/下"(1 ("上/下")) -> ()
                                n730 = Concatenate Strings("4楼" ("字符串"), "\r", "----" ("字符串")) -> (w569:string)
                                n731 = local write "6楼显示"(w569) -> ()
                                n732 = local write "1楼显示"(w569) -> ()
                                n733 = local write "2楼显示"(w569) -> ()
                                n734 = local write "3楼显示"(w569) -> ()
                                n735 = local write "4楼显示"(w569) -> ()
                                n736 = local write "5楼显示"(w569) -> ()
                                n737 = local write "电梯内显示"(w569) -> ()
                                }
                                frame #1 {
                                n738 = while {
                                stop <- w577 continue-if-true
                                n739 = local read "重量"() -> (w579:dbl)
                                n740 = Greater?(x=w579, y=1000.0 ("x")) -> (0:w577:bool)
                                n741 = local write "超重灯"(w577) -> ()
                                }
                                }
                                frame #2 {
                                n742 = while {
                                stop <- w580 continue-if-true
                                n743 = local read "开"() -> (w581:bool)
                                n744 = local read "开"() -> (w580:bool)
                                n745 = case shown="真" w581 {
                                frame False {
                                }
                                frame True {
                                n746 = local write "开"(FALSE ("常开")) -> ()
                                n747 = Wait (ms)(milliseconds to wait=u32 5000 ("等待时间（毫秒）")) -> ()  [unwired: 1 out]
                                }
                                }
                                }
                                }
                                frame #3 {
                                n748 = while {
                                stop <- w585 continue-if-true
                                n749 = local read "常开"() -> (w585:bool)
                                n750 = Wait (ms)(milliseconds to wait=u32 1 ("等待时间（毫秒）")) -> ()  [unwired: 1 out]
                                }
                                }
                                frame #4 {
                                w586 = FALSE ("1楼门")
                                n751 = local write "4楼门"(w586) -> ()
                                n752 = local write "电梯门"(w586) -> ()
                                n753 = local write "4上"(w586) -> ()
                                n754 = local write "关"(w586) -> ()
                                n755 = local write "开"(w586) -> ()
                                }
                                }
                                }
                                }
                                }
                              }
                            }
                            frame True {
                              n756 = flat-sequence {
                                tunnel: [FALSE] -> w588
                                frame #0 {
                                n757 = property class="Bool"() -> ("Top"=w594:i32)  [unwired: 2 in, 2 out]
                                n758 = Concatenate Strings("4楼" ("字符串"), "\r", "电梯下行" ("字符串")) -> (w589:string)
                                n759 = while {
                                shift-right: [w601] -> _
                                shift-left: w594 -> [w603]
                                stop <- w602 stop-if-true
                                n760 = Increment(x=w603) -> (x+1=w601:i32)
                                n761 = local write "上/下"(2 ("上/下")) -> ()
                                n762 = property class="Bool"("Top"=w601) -> ()  [unwired: 2 in, 2 out]
                                n763 = Equal?(x=w601, y=288) -> (x = y?=w602:bool)
                                n764 = local read "电梯快行"() -> (w597:bool)
                                n765 = Select(t=u32 1, s=w597, f=u32 25) -> (s? t:f=w598:u32)
                                n766 = Wait (ms)(milliseconds to wait=w598) -> ()  [unwired: 1 out]
                                }
                                n767 = local write "1楼显示"(w589) -> ()
                                n768 = local write "2楼显示"(w589) -> ()
                                n769 = local write "3楼显示"(w589) -> ()
                                n770 = local write "4楼显示"(w589) -> ()
                                n771 = local write "5楼显示"(w589) -> ()
                                n772 = local write "电梯内显示"(w589) -> ()
                                n773 = local write "6楼显示"(w589) -> ()
                                }
                              }
                            }
                          }
                        }
                      }
                    }
                    frame True {
                      n774 = flat-sequence {
                        tunnel: [FALSE] -> w604
                        frame #0 {
                          n775 = for {
                            N: 60 -> [_]
                            stop <- w610 stop-if-true
                            w612 = TRUE ("1楼门")
                            n776 = local read "关"() -> (w610:bool)
                            n777 = local write "电梯门"(w612) -> ()
                            n778 = local write "4楼门"(w612) -> ()
                            n779 = Wait (ms)(milliseconds to wait=u32 100 ("等待时间（毫秒）")) -> ()  [unwired: 1 out]
                          }
                          n780 = Concatenate Strings("4楼" ("字符串"), "\r", "----" ("字符串")) -> (w606:string)
                          n781 = local write "6楼显示"(w606) -> ()
                          n782 = local write "1楼显示"(w606) -> ()
                          n783 = local write "2楼显示"(w606) -> ()
                          n784 = local write "3楼显示"(w606) -> ()
                          n785 = local write "4楼显示"(w606) -> ()
                          n786 = local write "5楼显示"(w606) -> ()
                          n787 = local write "电梯内显示"(w606) -> ()
                        }
                        frame #1 {
                          n788 = while {
                            stop <- w613 continue-if-true
                            n789 = local read "重量"() -> (w615:dbl)
                            n790 = Greater?(x=w615, y=1000.0 ("x")) -> (0:w613:bool)
                            n791 = local write "超重灯"(w613) -> ()
                          }
                        }
                        frame #2 {
                          n792 = while {
                            stop <- w616 continue-if-true
                            n793 = local read "开"() -> (w617:bool)
                            n794 = local read "开"() -> (w616:bool)
                            n795 = case shown="真" w617 {
                              frame False {
                              }
                              frame True {
                                n796 = local write "开"(FALSE ("常开")) -> ()
                                n797 = Wait (ms)(milliseconds to wait=u32 5000 ("等待时间（毫秒）")) -> ()  [unwired: 1 out]
                              }
                            }
                          }
                        }
                        frame #3 {
                          n798 = while {
                            stop <- w621 continue-if-true
                            n799 = local read "常开"() -> (w621:bool)
                            n800 = Wait (ms)(milliseconds to wait=u32 1 ("等待时间（毫秒）")) -> ()  [unwired: 1 out]
                          }
                        }
                        frame #4 {
                          w622 = FALSE ("1楼门")
                          n801 = local write "4楼门"(w622) -> ()
                          n802 = local write "电梯门"(w622) -> ()
                          n803 = local write "4楼"(w622) -> ()
                          n804 = local write "4下"(w622) -> ()
                          n805 = local write "关"(w622) -> ()
                          n806 = local write "开"(w622) -> ()
                          n807 = local write "上/下"(2 ("上/下")) -> ()
                        }
                      }
                    }
                  }
                }
                frame 288 {
                  n808 = local read "3下"() -> (w628:bool)
                  n809 = local read "3楼"() -> (w627:bool)
                  n810 = Or(x=w628, y=w627) -> (x .or. y?=w626:bool)
                  n811 = case shown="假" w626 {
                    tunnel: [w632 w729] -> w625
                    frame False {
                      n812 = local read "5下"() -> (w629:bool)
                      n813 = local read "6楼"() -> (w630:bool)
                      n814 = local read "6下"() -> (w631:bool)
                      n815 = local read "5上"() -> (w644:bool)
                      n816 = local read "1楼"() -> (w643:bool)
                      n817 = local read "4下"() -> (w642:bool)
                      n818 = local read "2下"() -> (w641:bool)
                      n819 = local read "4上"() -> (w640:bool)
                      n820 = local read "3上"() -> (w639:bool)
                      n821 = local read "2上"() -> (w638:bool)
                      n822 = local read "5楼"() -> (w637:bool)
                      n823 = local read "1上"() -> (w636:bool)
                      n824 = local read "4楼"() -> (w635:bool)
                      n825 = local read "2楼"() -> (w634:bool)
                      n826 = Compound Arithmetic op=OR(w644, w643, w642, w641, w640, w639, w638, w637, w636, w635, w634, w631, w630, w629) -> (w633:bool)
                      n827 = case shown="真" w633 {
                        tunnel: [FALSE w652] -> w632
                        frame False {
                        }
                        frame True {
                          n828 = local read "1楼"() -> (w651:bool)
                          n829 = local read "1上"() -> (w650:bool)
                          n830 = local read "2下"() -> (w649:bool)
                          n831 = local read "2上"() -> (w648:bool)
                          n832 = local read "2楼"() -> (w646:bool)
                          n833 = Compound Arithmetic op=OR(w651, w650, w649, w648, w646) -> (w647:bool)
                          n834 = case shown="假" w647 {
                            tunnel: [w659 FALSE] -> w652
                            frame False {
                              n835 = local read "5上"() -> (w663:bool)
                              n836 = local read "4上"() -> (w662:bool)
                              n837 = local read "5楼"() -> (w661:bool)
                              n838 = local read "3上"() -> (w658:bool)
                              n839 = local read "4上"() -> (w657:bool)
                              n840 = local read "4下"() -> (w656:bool)
                              n841 = local read "5下"() -> (w653:bool)
                              n842 = local read "6楼"() -> (w654:bool)
                              n843 = local read "6下"() -> (w655:bool)
                              n844 = Compound Arithmetic op=OR(w663, w662, w661, w658, w657, w656, w655, w654, w653) -> (w660:bool)
                              n845 = case shown="真" w660 {
                                tunnel: [FALSE w665] -> w659
                                frame False {
                                }
                                frame True {
                                n846 = local read "3上"() -> (w666:bool)
                                n847 = case shown="真" w666 {
                                tunnel: [w676 w693] -> w665
                                frame False {
                                n848 = local read "4上"() -> (w675:bool)
                                n849 = local read "4楼"() -> (w674:bool)
                                n850 = local read "5楼"() -> (w673:bool)
                                n851 = local read "4下"() -> (w672:bool)
                                n852 = local read "5上"() -> (w670:bool)
                                n853 = local read "5下"() -> (w667:bool)
                                n854 = local read "6楼"() -> (w668:bool)
                                n855 = local read "6下"() -> (w669:bool)
                                n856 = Compound Arithmetic op=OR(w675, w674, w673, w672, w670, w669, w668, w667) -> (w671:bool)
                                n857 = case shown="假" w671 {
                                tunnel: [FALSE FALSE] -> w676
                                frame False {
                                }
                                frame True {
                                n858 = property class="Bool"() -> ("Top"=w683:i32)  [unwired: 2 in, 2 out]
                                n859 = Concatenate Strings("3楼" ("字符串"), "\r", "电梯上行" ("字符串")) -> (w679:string)
                                n860 = while {
                                shift-right: [w688] -> _
                                shift-left: w683 -> [w692]
                                stop <- w690 stop-if-true
                                n861 = Decrement(x=w692) -> (x-1=w688:i32)
                                n862 = local write "上/下"(1 ("上/下")) -> ()
                                n863 = Equal?(x=w688, y=144) -> (x = y?=w690:bool)
                                n864 = property class="Bool"("Top"=w688) -> ()  [unwired: 2 in, 2 out]
                                n865 = local read "电梯快行"() -> (w686:bool)
                                n866 = Select(t=u32 1, s=w686, f=u32 25) -> (s? t:f=w687:u32)
                                n867 = Wait (ms)(milliseconds to wait=w687) -> ()  [unwired: 1 out]
                                }
                                n868 = local write "电梯内显示"(w679) -> ()
                                n869 = local write "1楼显示"(w679) -> ()
                                n870 = local write "2楼显示"(w679) -> ()
                                n871 = local write "3楼显示"(w679) -> ()
                                n872 = local write "4楼显示"(w679) -> ()
                                n873 = local write "5楼显示"(w679) -> ()
                                }
                                }
                                }
                                frame True {
                                n874 = flat-sequence {
                                tunnel: [FALSE] -> w693
                                frame #0 {
                                n875 = local write "上/下"(1 ("上/下")) -> ()
                                n876 = for {
                                N: 60 -> [_]
                                stop <- w700 stop-if-true
                                w702 = TRUE ("1楼门")
                                n877 = local read "关"() -> (w700:bool)
                                n878 = local write "电梯门"(w702) -> ()
                                n879 = local write "3楼门"(w702) -> ()
                                n880 = Wait (ms)(milliseconds to wait=u32 100 ("等待时间（毫秒）")) -> ()  [unwired: 1 out]
                                }
                                n881 = Concatenate Strings("3楼" ("字符串"), "\r", "----" ("字符串")) -> (w695:string)
                                n882 = local write "1楼显示"(w695) -> ()
                                n883 = local write "2楼显示"(w695) -> ()
                                n884 = local write "3楼显示"(w695) -> ()
                                n885 = local write "4楼显示"(w695) -> ()
                                n886 = local write "5楼显示"(w695) -> ()
                                n887 = local write "电梯内显示"(w695) -> ()
                                n888 = local write "6楼显示"(w695) -> ()
                                }
                                frame #1 {
                                n889 = while {
                                stop <- w703 continue-if-true
                                n890 = local read "重量"() -> (w705:dbl)
                                n891 = Greater?(x=w705, y=1000.0 ("x")) -> (0:w703:bool)
                                n892 = local write "超重灯"(w703) -> ()
                                }
                                }
                                frame #2 {
                                n893 = while {
                                stop <- w706 continue-if-true
                                n894 = local read "开"() -> (w707:bool)
                                n895 = local read "开"() -> (w706:bool)
                                n896 = case shown="真" w707 {
                                frame False {
                                }
                                frame True {
                                n897 = local write "开"(FALSE ("常开")) -> ()
                                n898 = Wait (ms)(milliseconds to wait=u32 5000 ("等待时间（毫秒）")) -> ()  [unwired: 1 out]
                                }
                                }
                                }
                                }
                                frame #3 {
                                n899 = while {
                                stop <- w711 continue-if-true
                                n900 = local read "常开"() -> (w711:bool)
                                n901 = Wait (ms)(milliseconds to wait=u32 1 ("等待时间（毫秒）")) -> ()  [unwired: 1 out]
                                }
                                }
                                frame #4 {
                                w712 = FALSE ("1楼门")
                                n902 = local write "3楼门"(w712) -> ()
                                n903 = local write "电梯门"(w712) -> ()
                                n904 = local write "3上"(w712) -> ()
                                n905 = local write "关"(w712) -> ()
                                n906 = local write "开"(w712) -> ()
                                }
                                }
                                }
                                }
                                }
                              }
                            }
                            frame True {
                              n907 = property class="Bool"() -> ("Top"=w716:i32)  [unwired: 2 in, 2 out]
                              n908 = Concatenate Strings("3楼" ("字符串"), "\r", "电梯下行" ("字符串")) -> (w714:string)
                              n909 = while {
                                shift-right: [w726] -> _
                                shift-left: w716 -> [w728]
                                stop <- w725 stop-if-true
                                n910 = Increment(x=w728) -> (x+1=w726:i32)
                                n911 = Equal?(x=w726, y=432) -> (x = y?=w725:bool)
                                n912 = property class="Bool"("Top"=w726) -> ()  [unwired: 2 in, 2 out]
                                n913 = local read "电梯快行"() -> (w723:bool)
                                n914 = Select(t=u32 1, s=w723, f=u32 25) -> (s? t:f=w724:u32)
                                n915 = Wait (ms)(milliseconds to wait=w724) -> ()  [unwired: 1 out]
                              }
                              n916 = local write "上/下"(2 ("上/下")) -> ()
                              n917 = local write "1楼显示"(w714) -> ()
                              n918 = local write "2楼显示"(w714) -> ()
                              n919 = local write "3楼显示"(w714) -> ()
                              n920 = local write "4楼显示"(w714) -> ()
                              n921 = local write "5楼显示"(w714) -> ()
                              n922 = local write "电梯内显示"(w714) -> ()
                              n923 = local write "6楼显示"(w714) -> ()
                            }
                          }
                        }
                      }
                    }
                    frame True {
                      n924 = flat-sequence {
                        tunnel: [FALSE] -> w729
                        frame #0 {
                          n925 = for {
                            N: 60 -> [_]
                            stop <- w735 stop-if-true
                            w737 = TRUE ("1楼门")
                            n926 = local read "关"() -> (w735:bool)
                            n927 = local write "电梯门"(w737) -> ()
                            n928 = local write "3楼门"(w737) -> ()
                            n929 = Wait (ms)(milliseconds to wait=u32 100 ("等待时间（毫秒）")) -> ()  [unwired: 1 out]
                          }
                          n930 = Concatenate Strings("3楼" ("字符串"), "\r", "----" ("字符串")) -> (w731:string)
                          n931 = local write "1楼显示"(w731) -> ()
                          n932 = local write "2楼显示"(w731) -> ()
                          n933 = local write "3楼显示"(w731) -> ()
                          n934 = local write "4楼显示"(w731) -> ()
                          n935 = local write "5楼显示"(w731) -> ()
                          n936 = local write "电梯内显示"(w731) -> ()
                          n937 = local write "6楼显示"(w731) -> ()
                        }
                        frame #1 {
                          n938 = while {
                            stop <- w738 continue-if-true
                            n939 = local read "重量"() -> (w740:dbl)
                            n940 = Greater?(x=w740, y=1000.0 ("x")) -> (0:w738:bool)
                            n941 = local write "超重灯"(w738) -> ()
                          }
                        }
                        frame #2 {
                          n942 = while {
                            stop <- w741 continue-if-true
                            n943 = local read "开"() -> (w742:bool)
                            n944 = local read "开"() -> (w741:bool)
                            n945 = case shown="真" w742 {
                              frame False {
                              }
                              frame True {
                                n946 = local write "开"(FALSE ("常开")) -> ()
                                n947 = Wait (ms)(milliseconds to wait=u32 5000 ("等待时间（毫秒）")) -> ()  [unwired: 1 out]
                              }
                            }
                          }
                        }
                        frame #3 {
                          n948 = while {
                            stop <- w746 continue-if-true
                            n949 = local read "常开"() -> (w746:bool)
                            n950 = Wait (ms)(milliseconds to wait=u32 1 ("等待时间（毫秒）")) -> ()  [unwired: 1 out]
                          }
                        }
                        frame #4 {
                          w747 = FALSE ("1楼门")
                          n951 = local write "上/下"(2 ("上/下")) -> ()
                          n952 = local write "电梯门"(w747) -> ()
                          n953 = local write "3楼门"(w747) -> ()
                          n954 = local write "3楼"(w747) -> ()
                          n955 = local write "3下"(w747) -> ()
                          n956 = local write "开"(w747) -> ()
                          n957 = local write "关"(w747) -> ()
                        }
                      }
                    }
                  }
                }
                frame -144 {
                  n958 = local read "6楼"() -> (w752:bool)
                  n959 = local read "6下"() -> (w751:bool)
                  n960 = Or(x=w752, y=w751) -> (x .or. y?=w750:bool)
                  n961 = case shown="真" w750 {
                    tunnel: [w768 w785] -> _
                    frame False {
                      n962 = local read "4楼"() -> (w767:bool)
                      n963 = local read "3楼"() -> (w766:bool)
                      n964 = local read "2楼"() -> (w765:bool)
                      n965 = local read "1楼"() -> (w764:bool)
                      n966 = local read "1上"() -> (w763:bool)
                      n967 = local read "2上"() -> (w762:bool)
                      n968 = local read "3上"() -> (w761:bool)
                      n969 = local read "4上"() -> (w760:bool)
                      n970 = local read "4下"() -> (w759:bool)
                      n971 = local read "3下"() -> (w758:bool)
                      n972 = local read "2下"() -> (w756:bool)
                      n973 = local read "5上"() -> (w755:bool)
                      n974 = local read "5楼"() -> (w754:bool)
                      n975 = local read "5下"() -> (w753:bool)
                      n976 = Compound Arithmetic op=OR(w767, w766, w765, w764, w763, w762, w761, w760, w759, w758, w756, w755, w754, w753) -> (w757:bool)
                      n977 = case shown="真" w757 {
                        tunnel: [FALSE FALSE] -> w768
                        frame False {
                        }
                        frame True {
                          n978 = property class="Bool"() -> ("Top"=w775:i32)  [unwired: 2 in, 2 out]
                          n979 = while {
                            shift-right: [w782] -> _
                            shift-left: w775 -> [w781]
                            stop <- w783 stop-if-true
                            n980 = local read "电梯快行"() -> (w778:bool)
                            n981 = Increment(x=w781) -> (x+1=w782:i32)
                            n982 = local write "上/下"(2 ("上/下")) -> ()
                            n983 = property class="Bool"("Top"=w782) -> ()  [unwired: 2 in, 2 out]
                            n984 = Select(t=u32 1, s=w778, f=u32 25) -> (s? t:f=w779:u32)
                            n985 = Equal?(x=w782, y=0) -> (x = y?=w783:bool)
                            n986 = Wait (ms)(milliseconds to wait=w779) -> ()  [unwired: 1 out]
                          }
                          n987 = Concatenate Strings("6楼" ("字符串"), "\r", "电梯下行" ("字符串")) -> (w770:string)
                          n988 = local write "1楼显示"(w770) -> ()
                          n989 = local write "2楼显示"(w770) -> ()
                          n990 = local write "3楼显示"(w770) -> ()
                          n991 = local write "4楼显示"(w770) -> ()
                          n992 = local write "5楼显示"(w770) -> ()
                          n993 = local write "电梯内显示"(w770) -> ()
                          n994 = local write "6楼显示"(w770) -> ()
                        }
                      }
                    }
                    frame True {
                      n995 = flat-sequence {
                        tunnel: [FALSE] -> w785
                        frame #0 {
                          n996 = for {
                            N: 60 -> [_]
                            stop <- w791 stop-if-true
                            w793 = TRUE ("1楼门")
                            n997 = local read "关"() -> (w791:bool)
                            n998 = local write "电梯门"(w793) -> ()
                            n999 = local write "6楼门"(w793) -> ()
                            n1000 = Wait (ms)(milliseconds to wait=u32 100 ("等待时间（毫秒）")) -> ()  [unwired: 1 out]
                          }
                          n1001 = Concatenate Strings("6楼" ("字符串"), "\r", "----" ("字符串")) -> (w787:string)
                          n1002 = local write "6楼显示"(w787) -> ()
                          n1003 = local write "1楼显示"(w787) -> ()
                          n1004 = local write "2楼显示"(w787) -> ()
                          n1005 = local write "3楼显示"(w787) -> ()
                          n1006 = local write "4楼显示"(w787) -> ()
                          n1007 = local write "5楼显示"(w787) -> ()
                          n1008 = local write "电梯内显示"(w787) -> ()
                        }
                        frame #1 {
                          n1009 = while {
                            stop <- w794 continue-if-true
                            n1010 = local read "重量"() -> (w796:dbl)
                            n1011 = Greater?(x=w796, y=1000.0 ("x")) -> (0:w794:bool)
                            n1012 = local write "超重灯"(w794) -> ()
                          }
                        }
                        frame #2 {
                          n1013 = while {
                            stop <- w797 continue-if-true
                            n1014 = local read "开"() -> (w798:bool)
                            n1015 = case shown="真" w798 {
                              frame False {
                              }
                              frame True {
                                n1016 = local write "开"(FALSE ("常开")) -> ()
                                n1017 = Wait (ms)(milliseconds to wait=u32 5000 ("等待时间（毫秒）")) -> ()  [unwired: 1 out]
                              }
                            }
                            n1018 = local read "开"() -> (w797:bool)
                          }
                        }
                        frame #3 {
                          n1019 = while {
                            stop <- w802 continue-if-true
                            n1020 = local read "常开"() -> (w802:bool)
                            n1021 = Wait (ms)(milliseconds to wait=u32 1 ("等待时间（毫秒）")) -> ()  [unwired: 1 out]
                          }
                        }
                        frame #4 {
                          w803 = FALSE ("电梯门")
                          n1022 = local write "上/下"(2 ("上/下")) -> ()
                          n1023 = local write "6楼"(w803) -> ()
                          n1024 = local write "6下"(w803) -> ()
                          n1025 = local write "电梯门"(w803) -> ()
                          n1026 = local write "6楼门"(w803) -> ()
                          n1027 = local write "开"(w803) -> ()
                          n1028 = local write "关"(w803) -> ()
                        }
                      }
                    }
                  }
                }
                frame 432 {
                  n1029 = local read "2楼"() -> (w808:bool)
                  n1030 = local read "2下"() -> (w809:bool)
                  n1031 = Or(x=w809, y=w808) -> (x .or. y?=w807:bool)
                  n1032 = case shown="真" w807 {
                    tunnel: [w813 w913] -> w806
                    frame False {
                      n1033 = local read "5上"() -> (w825:bool)
                      n1034 = local read "1楼"() -> (w824:bool)
                      n1035 = local read "4下"() -> (w823:bool)
                      n1036 = local read "3下"() -> (w822:bool)
                      n1037 = local read "1上"() -> (w821:bool)
                      n1038 = local read "3上"() -> (w820:bool)
                      n1039 = local read "2上"() -> (w819:bool)
                      n1040 = local read "5楼"() -> (w818:bool)
                      n1041 = local read "4上"() -> (w817:bool)
                      n1042 = local read "4楼"() -> (w816:bool)
                      n1043 = local read "3楼"() -> (w815:bool)
                      n1044 = local read "6楼"() -> (w810:bool)
                      n1045 = local read "5下"() -> (w812:bool)
                      n1046 = local read "6下"() -> (w811:bool)
                      n1047 = Compound Arithmetic op=OR(w825, w824, w823, w822, w821, w820, w819, w818, w817, w816, w815, w812, w811, w810) -> (w814:bool)
                      n1048 = case shown="真" w814 {
                        tunnel: [FALSE w830] -> w813
                        frame False {
                        }
                        frame True {
                          n1049 = local read "1楼"() -> (w829:bool)
                          n1050 = local read "1上"() -> (w828:bool)
                          n1051 = Compound Arithmetic op=OR(w829, w828) -> (w827:bool)
                          n1052 = case shown="假" w827 {
                            tunnel: [w840 FALSE] -> w830
                            frame False {
                              n1053 = local read "6楼"() -> (w831:bool)
                              n1054 = local read "5上"() -> (w844:bool)
                              n1055 = local read "4楼"() -> (w843:bool)
                              n1056 = local read "5楼"() -> (w842:bool)
                              n1057 = local read "3上"() -> (w839:bool)
                              n1058 = local read "4上"() -> (w838:bool)
                              n1059 = local read "2上"() -> (w837:bool)
                              n1060 = local read "3楼"() -> (w836:bool)
                              n1061 = local read "3下"() -> (w835:bool)
                              n1062 = local read "4下"() -> (w834:bool)
                              n1063 = local read "5下"() -> (w833:bool)
                              n1064 = local read "6下"() -> (w832:bool)
                              n1065 = Compound Arithmetic op=OR(w844, w843, w842, w839, w838, w837, w836, w835, w834, w833, w832, w831) -> (w841:bool)
                              n1066 = case shown="真" w841 {
                                tunnel: [FALSE w846] -> w840
                                frame False {
                                }
                                frame True {
                                n1067 = local read "2上"() -> (w847:bool)
                                n1068 = case shown="真" w847 {
                                tunnel: [w860 w877] -> w846
                                frame False {
                                n1069 = local read "3上"() -> (w851:bool)
                                n1070 = local read "4上"() -> (w859:bool)
                                n1071 = local read "4楼"() -> (w858:bool)
                                n1072 = local read "5楼"() -> (w857:bool)
                                n1073 = local read "4下"() -> (w856:bool)
                                n1074 = local read "5上"() -> (w854:bool)
                                n1075 = local read "3楼"() -> (w853:bool)
                                n1076 = local read "3下"() -> (w852:bool)
                                n1077 = local read "6楼"() -> (w848:bool)
                                n1078 = local read "5下"() -> (w850:bool)
                                n1079 = local read "6下"() -> (w849:bool)
                                n1080 = Compound Arithmetic op=OR(w859, w858, w857, w856, w854, w853, w852, w851, w850, w849, w848) -> (w855:bool)
                                n1081 = case shown="真" w855 {
                                tunnel: [FALSE FALSE] -> w860
                                frame False {
                                }
                                frame True {
                                n1082 = property class="Bool"() -> ("Top"=w865:i32)  [unwired: 2 in, 2 out]
                                n1083 = Concatenate Strings("2楼" ("字符串"), "\r", "电梯上行" ("字符串")) -> (w862:string)
                                n1084 = while {
                                shift-right: [w875] -> _
                                shift-left: w865 -> [w876]
                                stop <- w873 stop-if-true
                                n1085 = Decrement(x=w876) -> (x-1=w875:i32)
                                n1086 = property class="Bool"("Top"=w875) -> ()  [unwired: 2 in, 2 out]
                                n1087 = local write "上/下"(1 ("上/下")) -> ()
                                n1088 = Equal?(x=w875, y=288) -> (x = y?=w873:bool)
                                n1089 = local read "电梯快行"() -> (w870:bool)
                                n1090 = Select(t=u32 1, s=w870, f=u32 25) -> (s? t:f=w871:u32)
                                n1091 = Wait (ms)(milliseconds to wait=w871) -> ()  [unwired: 1 out]
                                }
                                n1092 = local write "1楼显示"(w862) -> ()
                                n1093 = local write "2楼显示"(w862) -> ()
                                n1094 = local write "3楼显示"(w862) -> ()
                                n1095 = local write "4楼显示"(w862) -> ()
                                n1096 = local write "5楼显示"(w862) -> ()
                                n1097 = local write "6楼显示"(w862) -> ()
                                n1098 = local write "电梯内显示"(w862) -> ()
                                }
                                }
                                }
                                frame True {
                                n1099 = flat-sequence {
                                tunnel: [FALSE] -> w877
                                frame #0 {
                                n1100 = for {
                                N: 60 -> [_]
                                stop <- w884 stop-if-true
                                w886 = TRUE ("1楼门")
                                n1101 = local read "关"() -> (w884:bool)
                                n1102 = local write "电梯门"(w886) -> ()
                                n1103 = local write "2楼门"(w886) -> ()
                                n1104 = Wait (ms)(milliseconds to wait=u32 100 ("等待时间（毫秒）")) -> ()  [unwired: 1 out]
                                }
                                n1105 = local write "上/下"(1 ("上/下")) -> ()
                                n1106 = Concatenate Strings("2楼" ("字符串"), "\r", "----" ("字符串")) -> (w879:string)
                                n1107 = local write "1楼显示"(w879) -> ()
                                n1108 = local write "2楼显示"(w879) -> ()
                                n1109 = local write "3楼显示"(w879) -> ()
                                n1110 = local write "4楼显示"(w879) -> ()
                                n1111 = local write "5楼显示"(w879) -> ()
                                n1112 = local write "电梯内显示"(w879) -> ()
                                n1113 = local write "6楼显示"(w879) -> ()
                                }
                                frame #1 {
                                n1114 = while {
                                stop <- w887 continue-if-true
                                n1115 = local read "重量"() -> (w889:dbl)
                                n1116 = Greater?(x=w889, y=1000.0 ("x")) -> (0:w887:bool)
                                n1117 = local write "超重灯"(w887) -> ()
                                }
                                }
                                frame #2 {
                                n1118 = while {
                                stop <- w890 continue-if-true
                                n1119 = local read "开"() -> (w891:bool)
                                n1120 = case shown="真" w891 {
                                frame False {
                                }
                                frame True {
                                n1121 = local write "开"(FALSE ("常开")) -> ()
                                n1122 = Wait (ms)(milliseconds to wait=u32 5000 ("等待时间（毫秒）")) -> ()  [unwired: 1 out]
                                }
                                }
                                n1123 = local read "开"() -> (w890:bool)
                                }
                                }
                                frame #3 {
                                n1124 = while {
                                stop <- w895 continue-if-true
                                n1125 = local read "常开"() -> (w895:bool)
                                n1126 = Wait (ms)(milliseconds to wait=u32 1 ("等待时间（毫秒）")) -> ()  [unwired: 1 out]
                                }
                                }
                                frame #4 {
                                w896 = FALSE ("1楼门")
                                n1127 = local write "电梯门"(w896) -> ()
                                n1128 = local write "2楼门"(w896) -> ()
                                n1129 = local write "2上"(w896) -> ()
                                n1130 = local write "关"(w896) -> ()
                                n1131 = local write "开"(w896) -> ()
                                }
                                }
                                }
                                }
                                }
                              }
                            }
                            frame True {
                              n1132 = property class="Bool"() -> ("Top"=w900:i32)  [unwired: 2 in, 2 out]
                              n1133 = while {
                                shift-right: [w908] -> _
                                shift-left: w900 -> [w912]
                                stop <- w911 stop-if-true
                                n1134 = Increment(x=w912) -> (x+1=w908:i32)
                                n1135 = local write "上/下"(1 ("上/下")) -> ()
                                n1136 = property class="Bool"("Top"=w908) -> ()  [unwired: 2 in, 2 out]
                                n1137 = Equal?(x=w908, y=576) -> (x = y?=w911:bool)
                                n1138 = local read "电梯快行"() -> (w906:bool)
                                n1139 = Select(t=u32 1, s=w906, f=u32 25) -> (s? t:f=w907:u32)
                                n1140 = Wait (ms)(milliseconds to wait=w907) -> ()  [unwired: 1 out]
                              }
                              n1141 = Concatenate Strings("2楼" ("字符串"), "\r", "电梯下行" ("字符串")) -> (w898:string)
                              n1142 = local write "1楼显示"(w898) -> ()
                              n1143 = local write "2楼显示"(w898) -> ()
                              n1144 = local write "3楼显示"(w898) -> ()
                              n1145 = local write "4楼显示"(w898) -> ()
                              n1146 = local write "5楼显示"(w898) -> ()
                              n1147 = local write "电梯内显示"(w898) -> ()
                              n1148 = local write "6楼显示"(w898) -> ()
                            }
                          }
                        }
                      }
                    }
                    frame True {
                      n1149 = flat-sequence {
                        tunnel: [FALSE] -> w913
                        frame #0 {
                          n1150 = for {
                            N: 60 -> [_]
                            stop <- w919 stop-if-true
                            w921 = TRUE ("1楼门")
                            n1151 = local read "关"() -> (w919:bool)
                            n1152 = local write "电梯门"(w921) -> ()
                            n1153 = local write "2楼门"(w921) -> ()
                            n1154 = Wait (ms)(milliseconds to wait=u32 100 ("等待时间（毫秒）")) -> ()  [unwired: 1 out]
                          }
                          n1155 = Concatenate Strings("2楼" ("字符串"), "\r", "----" ("字符串")) -> (w915:string)
                          n1156 = local write "1楼显示"(w915) -> ()
                          n1157 = local write "2楼显示"(w915) -> ()
                          n1158 = local write "3楼显示"(w915) -> ()
                          n1159 = local write "4楼显示"(w915) -> ()
                          n1160 = local write "5楼显示"(w915) -> ()
                          n1161 = local write "电梯内显示"(w915) -> ()
                          n1162 = local write "6楼显示"(w915) -> ()
                        }
                        frame #1 {
                          n1163 = while {
                            stop <- w922 continue-if-true
                            n1164 = local read "重量"() -> (w924:dbl)
                            n1165 = Greater?(x=w924, y=1000.0 ("x")) -> (0:w922:bool)
                            n1166 = local write "超重灯"(w922) -> ()
                          }
                        }
                        frame #2 {
                          n1167 = while {
                            stop <- w925 continue-if-true
                            n1168 = local read "开"() -> (w926:bool)
                            n1169 = local read "开"() -> (w925:bool)
                            n1170 = case shown="真" w926 {
                              frame False {
                              }
                              frame True {
                                n1171 = local write "开"(FALSE ("常开")) -> ()
                                n1172 = Wait (ms)(milliseconds to wait=u32 5000 ("等待时间（毫秒）")) -> ()  [unwired: 1 out]
                              }
                            }
                          }
                        }
                        frame #3 {
                          n1173 = while {
                            stop <- w930 continue-if-true
                            n1174 = local read "常开"() -> (w930:bool)
                            n1175 = Wait (ms)(milliseconds to wait=u32 1 ("等待时间（毫秒）")) -> ()  [unwired: 1 out]
                          }
                        }
                        frame #4 {
                          w931 = FALSE ("1楼门")
                          n1176 = local write "上/下"(2 ("上/下")) -> ()
                          n1177 = local write "电梯门"(w931) -> ()
                          n1178 = local write "2楼门"(w931) -> ()
                          n1179 = local write "2楼"(w931) -> ()
                          n1180 = local write "2下"(w931) -> ()
                          n1181 = local write "关"(w931) -> ()
                          n1182 = local write "开"(w931) -> ()
                        }
                      }
                    }
                  }
                }
                frame 0 {
                  n1183 = local read "5下"() -> (w937:bool)
                  n1184 = local read "5楼"() -> (w936:bool)
                  n1185 = Or(x=w937, y=w936) -> (x .or. y?=w934:bool)
                  n1186 = case shown="真" w934 {
                    tunnel: [w950 w1010] -> w935
                    frame False {
                      n1187 = local read "4楼"() -> (w949:bool)
                      n1188 = local read "3楼"() -> (w948:bool)
                      n1189 = local read "2楼"() -> (w947:bool)
                      n1190 = local read "1楼"() -> (w946:bool)
                      n1191 = local read "1上"() -> (w945:bool)
                      n1192 = local read "2上"() -> (w944:bool)
                      n1193 = local read "3上"() -> (w943:bool)
                      n1194 = local read "4上"() -> (w942:bool)
                      n1195 = local read "4下"() -> (w941:bool)
                      n1196 = local read "3下"() -> (w940:bool)
                      n1197 = local read "2下"() -> (w939:bool)
                      n1198 = Compound Arithmetic op=OR(w949, w948, w947, w946, w945, w944, w943, w942, w941, w940, w939) -> (w938:bool)
                      n1199 = case shown="假" w938 {
                        tunnel: [w951 FALSE] -> w950
                        frame False {
                          n1200 = local read "5上"() -> (w952:bool)
                          n1201 = case shown="真" w952 {
                            tunnel: [w953 w973] -> w951
                            frame False {
                              n1202 = local read "6下"() -> (w956:bool)
                              n1203 = local read "6楼"() -> (w955:bool)
                              n1204 = Or(x=w956, y=w955) -> (x .or. y?=w954:bool)
                              n1205 = case shown="真" w954 {
                                tunnel: [FALSE FALSE] -> w953
                                frame False {
                                }
                                frame True {
                                n1206 = property class="Bool"() -> ("Top"=w963:i32)  [unwired: 2 in, 2 out]
                                n1207 = while {
                                shift-right: [w970] -> _
                                shift-left: w963 -> [w969]
                                stop <- w971 stop-if-true
                                n1208 = local read "电梯快行"() -> (w966:bool)
                                n1209 = Increment(x=w969) -> (x+1=w970:i32)
                                n1210 = local write "上/下"(2 ("上/下")) -> ()
                                n1211 = Select(t=u32 1, s=w966, f=u32 25) -> (s? t:f=w967:u32)
                                n1212 = property class="Bool"("Top"=w970) -> ()  [unwired: 2 in, 2 out]
                                n1213 = Equal?(x=w970, y=-144) -> (x = y?=w971:bool)
                                n1214 = Wait (ms)(milliseconds to wait=w967) -> ()  [unwired: 1 out]
                                }
                                n1215 = Concatenate Strings("5楼" ("字符串"), "\r", "电梯下行" ("字符串")) -> (w959:string)
                                n1216 = local write "1楼显示"(w959) -> ()
                                n1217 = local write "2楼显示"(w959) -> ()
                                n1218 = local write "3楼显示"(w959) -> ()
                                n1219 = local write "4楼显示"(w959) -> ()
                                n1220 = local write "5楼显示"(w959) -> ()
                                n1221 = local write "电梯内显示"(w959) -> ()
                                n1222 = local write "6楼显示"(w959) -> ()
                                }
                              }
                            }
                            frame True {
                              n1223 = flat-sequence {
                                tunnel: [FALSE] -> _
                                tunnel: [FALSE] -> w973
                                frame #0 {
                                n1224 = for {
                                N: 60 -> [_]
                                stop <- w979 stop-if-true
                                w981 = TRUE ("1楼门")
                                n1225 = local read "关"() -> (w979:bool)
                                n1226 = local write "电梯门"(w981) -> ()
                                n1227 = local write "5楼门"(w981) -> ()
                                n1228 = Wait (ms)(milliseconds to wait=u32 100 ("等待时间（毫秒）")) -> ()  [unwired: 1 out]
                                }
                                n1229 = Concatenate Strings("5楼" ("字符串"), "\r", "----" ("字符串")) -> (w975:string)
                                n1230 = local write "6楼显示"(w975) -> ()
                                n1231 = local write "1楼显示"(w975) -> ()
                                n1232 = local write "2楼显示"(w975) -> ()
                                n1233 = local write "3楼显示"(w975) -> ()
                                n1234 = local write "4楼显示"(w975) -> ()
                                n1235 = local write "5楼显示"(w975) -> ()
                                n1236 = local write "电梯内显示"(w975) -> ()
                                }
                                frame #1 {
                                n1237 = while {
                                stop <- w982 continue-if-true
                                n1238 = local read "重量"() -> (w984:dbl)
                                n1239 = Greater?(x=w984, y=1000.0 ("x")) -> (0:w982:bool)
                                n1240 = local write "超重灯"(w982) -> ()
                                }
                                }
                                frame #2 {
                                n1241 = while {
                                stop <- w985 continue-if-true
                                n1242 = local read "开"() -> (w986:bool)
                                n1243 = case shown="真" w986 {
                                frame False {
                                }
                                frame True {
                                n1244 = local write "开"(FALSE ("常开")) -> ()
                                n1245 = Wait (ms)(milliseconds to wait=u32 5000 ("等待时间（毫秒）")) -> ()  [unwired: 1 out]
                                }
                                }
                                n1246 = local read "开"() -> (w985:bool)
                                }
                                }
                                frame #3 {
                                n1247 = while {
                                stop <- w990 continue-if-true
                                n1248 = local read "常开"() -> (w990:bool)
                                n1249 = Wait (ms)(milliseconds to wait=u32 1 ("等待时间（毫秒）")) -> ()  [unwired: 1 out]
                                }
                                }
                                frame #4 {
                                w991 = FALSE ("电梯门")
                                n1250 = local write "上/下"(1 ("上/下")) -> ()
                                n1251 = local write "电梯门"(w991) -> ()
                                n1252 = local write "5楼门"(w991) -> ()
                                n1253 = local write "5上"(w991) -> ()
                                n1254 = local write "关"(w991) -> ()
                                n1255 = local write "开"(w991) -> ()
                                }
                              }
                            }
                          }
                        }
                        frame True {
                          n1256 = property class="Bool"() -> ("Top"=w1000:i32)  [unwired: 2 in, 2 out]
                          n1257 = while {
                            shift-right: [w1007] -> _
                            shift-left: w1000 -> [w1006]
                            stop <- w1008 stop-if-true
                            n1258 = local read "电梯快行"() -> (w1003:bool)
                            n1259 = Increment(x=w1006) -> (x+1=w1007:i32)
                            n1260 = local write "上/下"(2 ("上/下")) -> ()
                            n1261 = property class="Bool"("Top"=w1007) -> ()  [unwired: 2 in, 2 out]
                            n1262 = Select(t=u32 1, s=w1003, f=u32 25) -> (s? t:f=w1004:u32)
                            n1263 = Equal?(x=w1007, y=144) -> (x = y?=w1008:bool)
                            n1264 = Wait (ms)(milliseconds to wait=w1004) -> ()  [unwired: 1 out]
                          }
                          n1265 = Concatenate Strings("5楼" ("字符串"), "\r", "电梯下行" ("字符串")) -> (w995:string)
                          n1266 = local write "1楼显示"(w995) -> ()
                          n1267 = local write "2楼显示"(w995) -> ()
                          n1268 = local write "3楼显示"(w995) -> ()
                          n1269 = local write "4楼显示"(w995) -> ()
                          n1270 = local write "5楼显示"(w995) -> ()
                          n1271 = local write "电梯内显示"(w995) -> ()
                          n1272 = local write "6楼显示"(w995) -> ()
                        }
                      }
                    }
                    frame True {
                      n1273 = flat-sequence {
                        tunnel: [FALSE] -> w1010
                        frame #0 {
                          n1274 = Concatenate Strings("5楼" ("字符串"), "\r", "----" ("字符串")) -> (w1012:string)
                          n1275 = for {
                            N: 60 -> [_]
                            stop <- w1016 stop-if-true
                            w1018 = TRUE ("1楼门")
                            n1276 = local read "关"() -> (w1016:bool)
                            n1277 = local write "电梯门"(w1018) -> ()
                            n1278 = local write "5楼门"(w1018) -> ()
                            n1279 = Wait (ms)(milliseconds to wait=u32 100 ("等待时间（毫秒）")) -> ()  [unwired: 1 out]
                          }
                          n1280 = local write "1楼显示"(w1012) -> ()
                          n1281 = local write "2楼显示"(w1012) -> ()
                          n1282 = local write "3楼显示"(w1012) -> ()
                          n1283 = local write "4楼显示"(w1012) -> ()
                          n1284 = local write "5楼显示"(w1012) -> ()
                          n1285 = local write "电梯内显示"(w1012) -> ()
                          n1286 = local write "6楼显示"(w1012) -> ()
                        }
                        frame #1 {
                          n1287 = while {
                            stop <- w1019 continue-if-true
                            n1288 = local read "重量"() -> (w1021:dbl)
                            n1289 = Greater?(x=w1021, y=1000.0 ("x")) -> (0:w1019:bool)
                            n1290 = local write "超重灯"(w1019) -> ()
                          }
                        }
                        frame #2 {
                          n1291 = while {
                            stop <- w1022 continue-if-true
                            n1292 = local read "开"() -> (w1023:bool)
                            n1293 = local read "开"() -> (w1022:bool)
                            n1294 = case shown="真" w1023 {
                              frame False {
                              }
                              frame True {
                                n1295 = local write "开"(FALSE ("常开")) -> ()
                                n1296 = Wait (ms)(milliseconds to wait=u32 5000 ("等待时间（毫秒）")) -> ()  [unwired: 1 out]
                              }
                            }
                          }
                        }
                        frame #3 {
                          n1297 = while {
                            stop <- w1027 continue-if-true
                            n1298 = local read "常开"() -> (w1027:bool)
                            n1299 = Wait (ms)(milliseconds to wait=u32 1 ("等待时间（毫秒）")) -> ()  [unwired: 1 out]
                          }
                        }
                        frame #4 {
                          w1028 = FALSE ("电梯门")
                          n1300 = local write "上/下"(2 ("上/下")) -> ()
                          n1301 = local write "电梯门"(w1028) -> ()
                          n1302 = local write "5楼门"(w1028) -> ()
                          n1303 = local write "5下"(w1028) -> ()
                          n1304 = local write "5楼"(w1028) -> ()
                          n1305 = local write "关"(w1028) -> ()
                          n1306 = local write "开"(w1028) -> ()
                        }
                      }
                    }
                  }
                }
              }
            }
          }
        }
      }
    }
  }
